vi "Main.vi"() -> ()   [LabVIEW 2020]
doc: "This Continuous Measurement sample project is based on the Queued Message Handler template.\n\nThe Event Handling Loop generates messages based on user interface actions.\n\nThe Message Handling Loop processes messages generated by the Event Handling Loop, or by other messages. There are also Acquisition and Logging message handling loop subVIs, and a chart updating loop."
uses:
  Settings/Settings.ctl
  Acquisition/Hardware Configuration.ctl
  Logging/Logging Configuration.ctl
  controls/UI Data.ctl
  controls/UI State.ctl
  support/Message Queue/Enqueue Message (Single).vi
  <vilib>/Utility/error.llb/Error Cluster From Error Code.vi
  <vilib>/ErrorRing/Error Ring.xnode
  Acquisition/Acquisition.lvlib
  Logging/Logging.lvlib
  Settings/Settings.lvlib
  support/User Event - Stop/User Event - Stop.lvlib
  support/Message Queue/Message Queue.lvlib
  2840X Software Library/Copy of BK PRECISION 2840 Folder/Copy of BK PRECISION 2840.lvlib
  Settings/Settings Dialog.vi
panel:
  in  "Stat In":T1
  out "Tab Ref":refnum<vi>
  out "Trigger Ref":refnum<vi>
  out "COMP Ref":refnum<vi>
  in  "Disconnect":bool
  in  "Connect":bool=TRUE
  out "BIN NO. Ref":refnum<vi>
  out "BIN No.State":bool
  out "BIN State Value":i32
  out "Tolerance New Val":dbl
  out "% Tolerance Ref":refnum<vi>
  out "Nom New Val":dbl
  out "Nominal REF":refnum<vi>
  out "BIN Event Ref":refnum<vi>
  out "Stat Ref":refnum<vi>
  out "Meas Ctl":refnum<vi>
  in  "Meas Tab":enum32{"Measure"}(tab)
  in  "Manual Range":u16(ring)=4 items=["20 m ", "200 m", "2", "20", "200", "2 K", "20 K", "100 K", "1 M", "10 M", "100 M"]
  in  "Auto Range":bool=TRUE
  in  "Function":i32(ring) items=["Resistance", "Resistance and Temperature", "Temperature", "LPR", "LPRT"]
  in  "Aperture":i32(ring)=2 items=["FAST", "MED", "SLOW1", "SLOW2"]
  in  "Average Readings":i32=1 min=1 max=255 step=10
  in  "Trigger Source":u16(ring) items=["Internal", "Manual", "External", "Software (Bus)"]
  in  "Auto Delay":bool=TRUE
  in  "Manual Trigger Delay":dbl=5.0 min=0.0 max=9.999 step=1.0
  in  "Trigger 2":bool
  out "Res":dbl format="%#_6p"
  out "Temp":dbl
  out "Function":string
  out "Meas Color Box":u32(colorbox)=11347 caption="Color Box"
  in  "Tab Control":enum32{"Statistics", "BIN", "Comparator"}(tab)
  out "In Samlpe Count":i32 format="%.0p"
  out "Sample Count":i32 format="%.0p"
  out "MAX":dbl format="%#_6p"
  out "MAX Index":i32 format="%.0p"
  out "MIN":dbl format="%#_6p"
  out "MIN Index":i32 format="%.0p"
  out "HIGH":i32 format="%.0p"
  out "IN":i32 format="%.0p"
  out "LOW":i32 format="%.0p"
  out "MEAS Error":i32 format="%.0p"
  out "Deviation":dbl format="%#_6p"
  out "Variance":dbl format="%#_6p"
  out "Cp":dbl format="%#_6p"
  out "Cpk":i32 format="%.0p"
  in  "Trigger":bool
  in  "Trigger Count":i32=1 min=1 max=250
  in  "Statistics Clear":bool
  in  "Deviation":dbl caption="% Deviation" min=0.0 max=99.999 step=1.0 format="%#_6p"
  in  "Nominal":dbl min=0.0 max=2200000.0 step=1000.0 format="%#_6p"
  in  "State":bool
  in  "Statistics Mode":u16(ring) items=["Percent Error", "Absolute"]
  out "Mean":dbl format="%#_6p"
  out "Stat Color Box":u32(colorbox)=3684408 caption="Color Box"
  in  "BIN State":bool caption="State"
  in  "Beeper Mode":u16(ring) items=["Off", "Beep when Pass", "Beep when Failed"]
  in  "BIN Mode":u16(ring) items=["Tolerance", "Absolute"]
  in  "% Tolerance":T2={"BIN 1"=1.0, "BIN 2"=1.0, "BIN 3"=1.0, "BIN 4"=1.0, "BIN 5"=1.0, "BIN 6"=1.0, "BIN 7"=1.0, "BIN 8"=1.0, "BIN 9"=1.0, "BIN 10"=1.0} {"BIN 10" min=1.0 step=100.0 format="%#_6p"; "BIN 9" min=1.0 step=100.0 format="%#_6p"; "BIN 8" min=1.0 step=100.0 format="%#_6p"; "BIN 7" min=1.0 step=100.0 format="%#_6p"; "BIN 6" min=1.0 step=100.0 format="%#_6p"; "BIN 5" min=1.0 step=100.0 format="%#_6p"; "BIN 4" min=1.0 step=100.0 format="%#_6p"; "BIN 3" min=1.0 step=100.0 format="%#_6p"; "BIN 2" min=1.0 step=100.0 format="%#_6p"; "BIN 1" min=1.0 step=100.0 format="%#_6p"}
  in  "Nominal":T2 {"BIN 10" step=100.0 format="%#_6p"; "BIN 9" step=100.0 format="%#_6p"; "BIN 8" step=100.0 format="%#_6p"; "BIN 7" step=100.0 format="%#_6p"; "BIN 6" step=100.0 format="%#_6p"; "BIN 5" step=100.0 format="%#_6p"; "BIN 4" step=100.0 format="%#_6p"; "BIN 3" step=100.0 format="%#_6p"; "BIN 2" step=100.0 format="%#_6p"; "BIN 1" step=100.0 format="%#_6p"}
  in  "BIN No.":T3
  out "BIN Display":T3
  in  "Comparator Lower":dbl caption="% Tolerance" min=0.0 max=2200000.0 step=1000.0 format="%#_6p"
  in  "Comparator Upper":dbl caption="Nominal" min=0.0 max=2200000.0 step=1000.0 format="%#_6p"
  in  "Comparator Clear":bool
  in  "Comparator Mode":u16(ring) items=["Percent Error", "Absolute"]
  in  "Comparator Beeper":u16(ring) items=["OFF", "NG", "GD"]
  in  "COMP State":bool caption="State"
  out "Comp":string
  out "HI :":i32
  out "LO :":i32
  out "IN :":i32
  out "TOT :":i32
  out "Color Box 3":u32(colorbox)=3684408 caption="Color Box"
  out "Model":string
  out "SN":string
  out "FW Ver.":string
  in  "Settings":bool
  in  "Start":bool
  in  "Stop":bool
  out "Status":string
  in  "Exit":bool
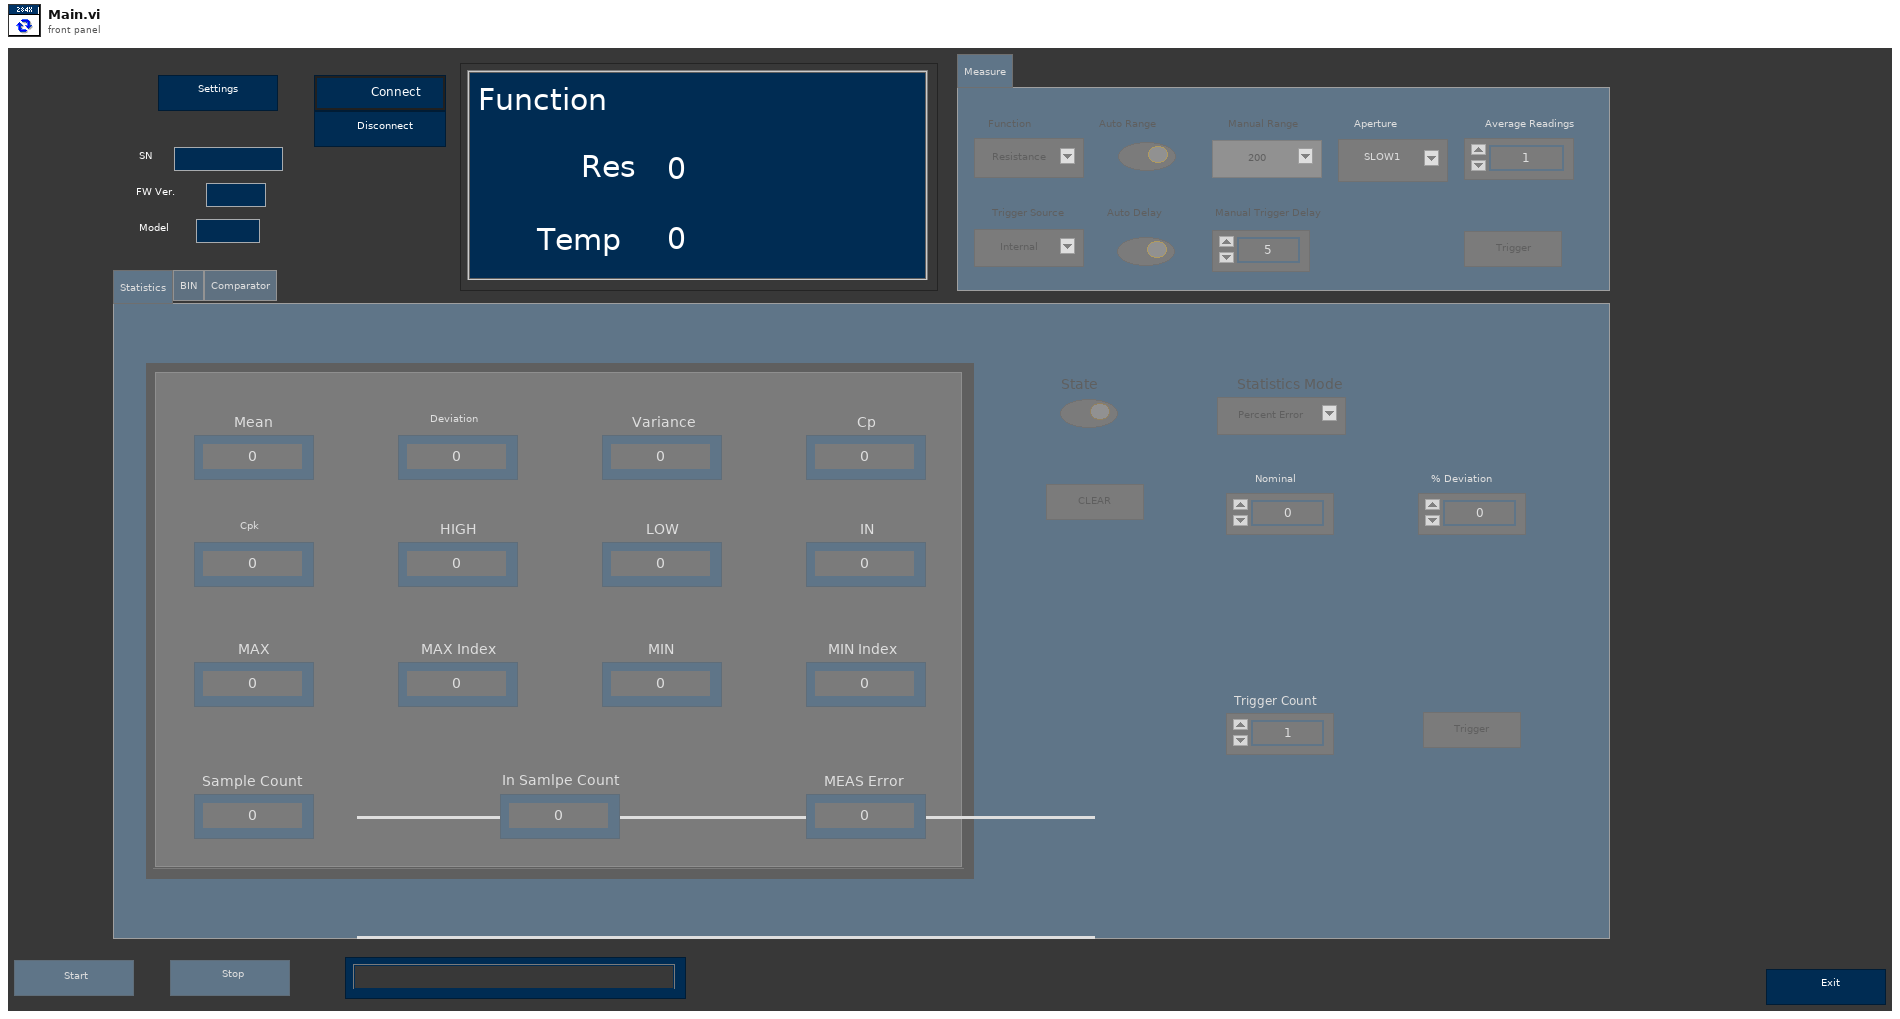
[diagram p1: front panel]
types:
  T1 = cluster{"Sample Count":i32, "IN Sample Count":i32, "Mean":dbl, "MAX":dbl, "MAX Index":i32, "MIN":dbl, "MIN Index":i32, "HIGH":i32, "IN":i32, "LOW":i32, "MEAS Error":i32, "Deviation":dbl, "Variance":dbl, "Cp":dbl, "CpK":i32}
  T2 = cluster{"BIN 1":dbl, "BIN 2":dbl, "BIN 3":dbl, "BIN 4":dbl, "BIN 5":dbl, "BIN 6":dbl, "BIN 7":dbl, "BIN 8":dbl, "BIN 9":dbl, "BIN 10":dbl}
  T3 = cluster{"BIN 1":bool, "BIN 2":bool, "BIN 3":bool, "BIN 4":bool, "BIN 5":bool, "BIN 6":bool, "BIN 7":bool, "BIN 8":bool, "BIN 9":bool, "BIN 10":bool}
  T4 = cluster{"Resistance":dbl, "Temp":dbl, "Function":string}
  T5 = cluster{"Result":string, "Total":i32, " IN":i32, "High":i32, "Low":i32}
  T6 = typedef "UI State.ctl" = enum16{"Idle", "Acquiring and Logging", "Waiting for Exit", "Waiting for Exit (Acq Stopped)", "Waiting for Exit (Log Stopped)", "Waiting for Stop", "Waiting for Stop (Acq Stopped)", "Waiting for Stop (Log Stopped)"}
  T7 = typedef "UI Data.ctl" = cluster{"Start Ref":refnum<vi>, "Stop Ref":refnum<vi>, "Settings Ref":refnum<vi>, "Exit Ref":refnum<vi>, "Status Ref":refnum<vi>, "Meas Trig":refnum<vi>, "Stat Trig":refnum<vi>, "COMP Trig":refnum<vi>, "COMP Mode":refnum<vi>, "COMP Beeper":refnum<vi>, "COMP  Tol":refnum<vi>, "COMP  Nom":refnum<vi>}
  T8 = typedef "Settings.lvlib/Settings.ctl" = cluster{"Hardware Configuration":T9, "Logging Configuration":T10}
  T9 = typedef "Acquisition.lvlib/Hardware Configuration.ctl" = cluster{"Inst.":refnum<visa-resource-name>, "Serial Configuration":cluster{"Baud Rate":u32, "Parity":u16, "Data Bits":u16, "Stop Bits":u16, "Flow Control":u16}, "Reset":bool, "Trigger Count":i32, "BIN State":bool, "COMP State":bool, "Trigger Source":u16, "Stat State ":bool}
  T10 = typedef "Logging.lvlib/Logging Configuration.ctl" = cluster{"*IDN?":string, "File Path":path, "File Path Ref":refnum<file>}
  T11 = typedef "Message Queue.lvlib/All Message Queues.ctl" = cluster{"UI":refnum<queue>, "Acquisition":refnum<queue>, "Logging":refnum<queue>}
  T12 = enum8{"Enabled", "Disabled", "Disabled and Grayed Out"}
  T13 = cluster{"Baud Rate":u32, "Parity":u16, "Data Bits":u16, "Stop Bits":u16, "Flow Control":u16}
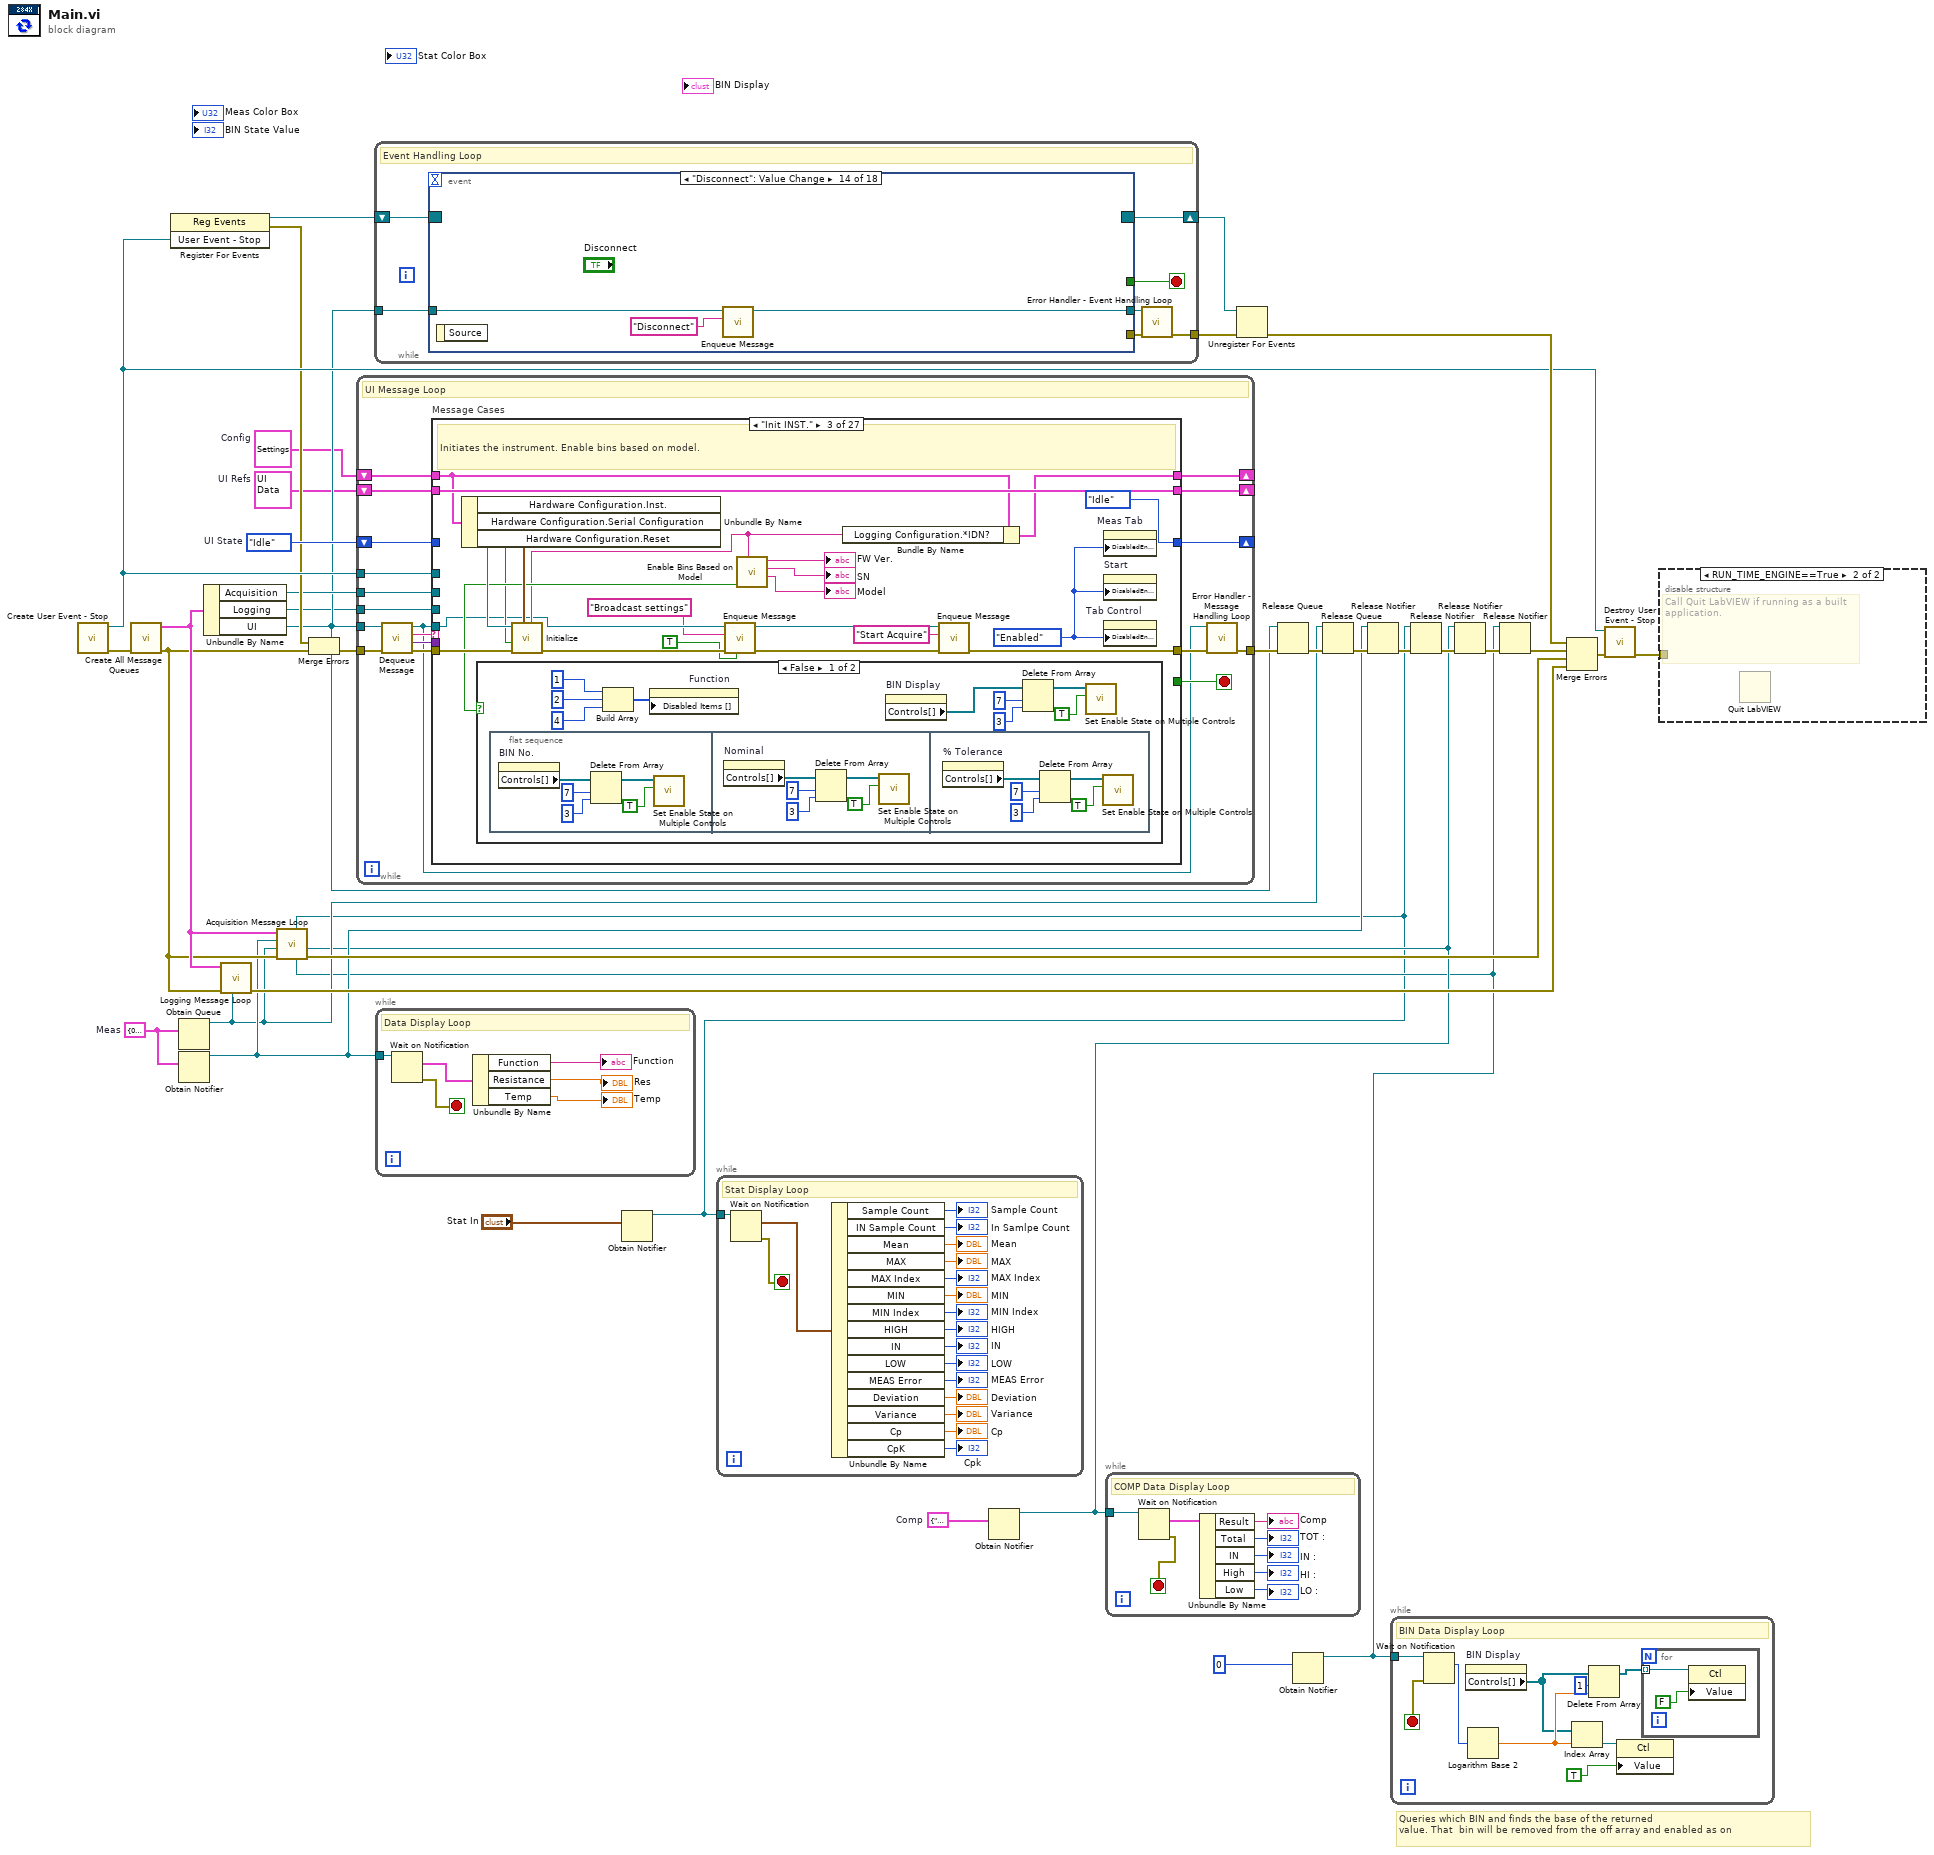
[diagram p0: block diagram]
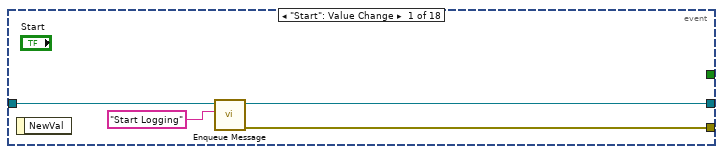
[diagram p3: hidden frame]
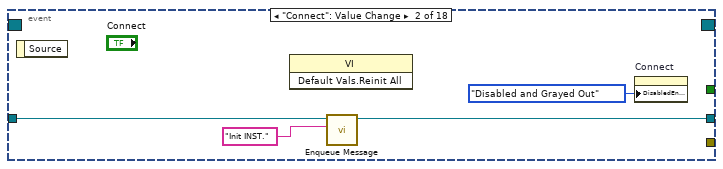
[diagram p4: hidden frame]
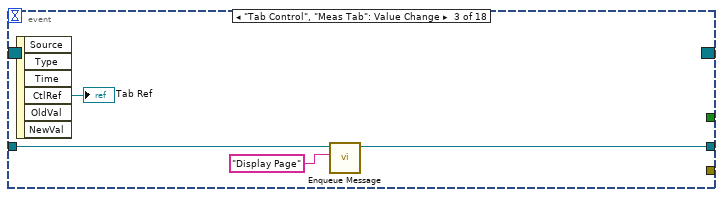
[diagram p5: hidden frame]
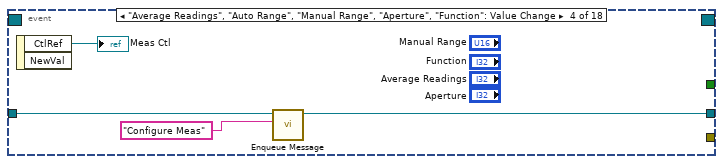
[diagram p6: hidden frame]
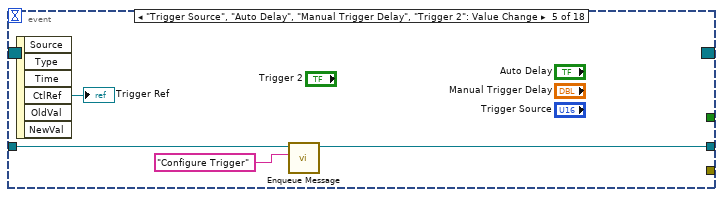
[diagram p7: hidden frame]
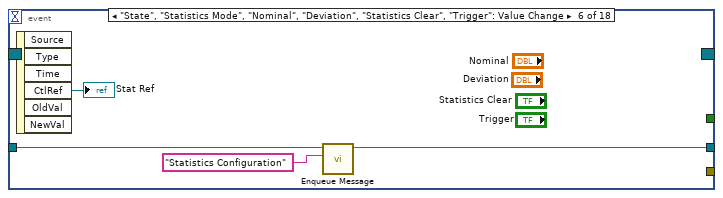
[diagram p8: hidden frame]
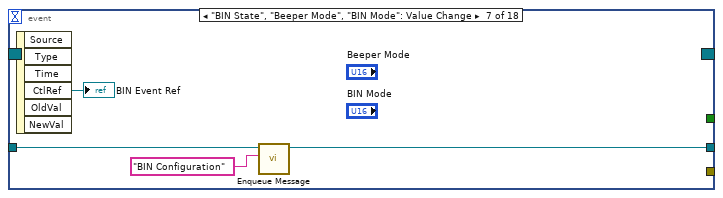
[diagram p9: hidden frame]
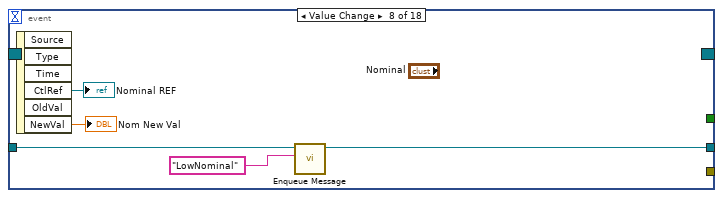
[diagram p10: hidden frame]
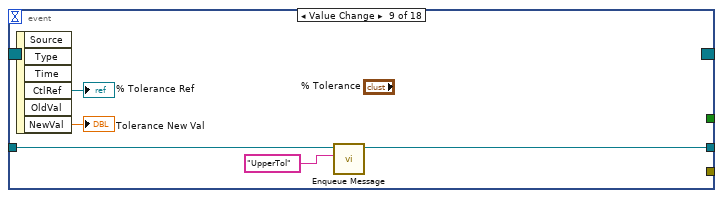
[diagram p11: hidden frame]
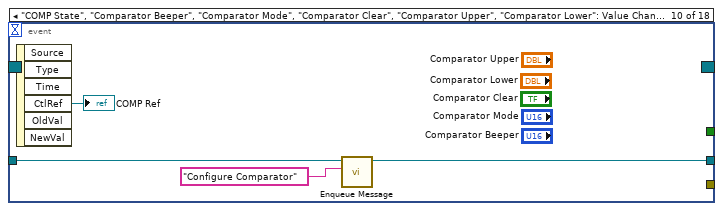
[diagram p12: hidden frame]
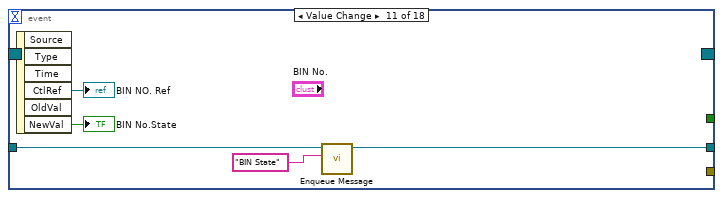
[diagram p13: hidden frame]
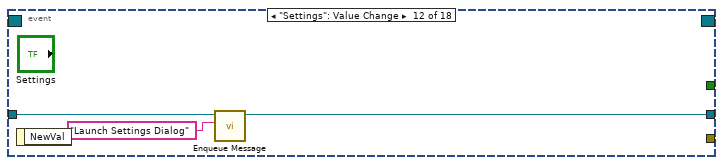
[diagram p14: hidden frame]
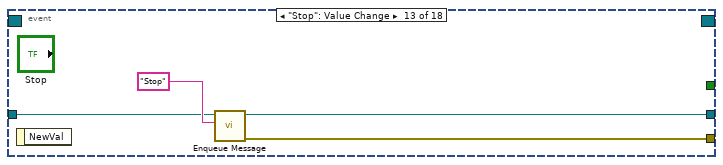
[diagram p15: hidden frame]
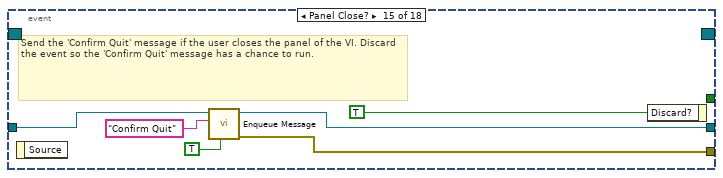
[diagram p16: hidden frame]
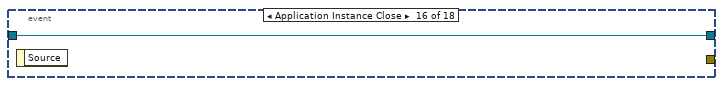
[diagram p17: hidden frame]
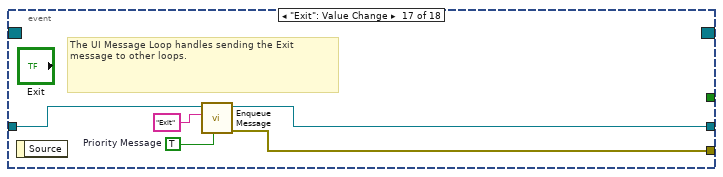
[diagram p18: hidden frame]
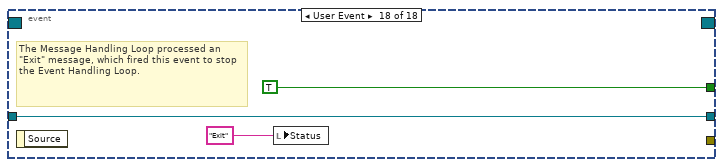
[diagram p19: hidden frame]
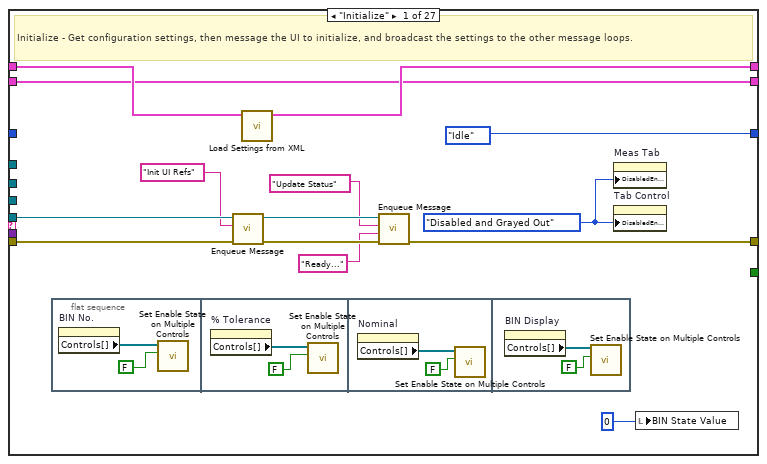
[diagram p20: hidden frame]
diagram:
  w1 = T4 {"Resistance"=0.0, "Temp"=0.0, "Function"=""}  # Meas
  w10 = T5 {"Result"="", "Total"=0, " IN"=0, "High"=0, "Low"=0}  # Comp
  w27 = UI_State."Idle"  # UI State
  w15 = T7 {"Start Ref"=refnum, "Stop Ref"=refnum, "Settings Ref"=refnum, "Exit Ref"=refnum, "Status Ref"=refnum, "Meas Trig"=refnum, "Stat Trig"=refnum, "COMP Trig"=refnum, "COMP Mode"=refnum, "COMP Beeper"=refnum, "COMP  Tol"=refnum, "COMP  Nom"=refnum}  # UI Refs
  w14 = T8 {"Hardware Configuration"={"Inst."="", "Serial Configuration"={"Baud Rate"=0, "Parity"=0, "Data Bits"=8, "Stop Bits"=10, "Flow Control"=0}, "Reset"=FALSE, "Trigger Count"=1, "BIN State"=FALSE, "COMP State"=FALSE, "Trigger Source"=0, "Stat State "=FALSE}, "Logging Configuration"={"*IDN?"="", "File Path"=path "", "File Path Ref"=refnum}}  # Config
  # "Queries which BIN and finds the base of the returned\nvalue. That  bin will be removed from the off array and enabled as on"
  n1 = call "Create User Event - Stop.vi"() -> ("error out"=w33:errorcluster, "User Event - Stop"=w21:refnum<user-event>)  [unwired: 10 in]
  n2 = call "Create All Message Queues.vi"("error in (no error)"=w33) -> ("error out"=w30:errorcluster, "Message Queues out"=w32:T11)  [unwired: 9 in]
  n3 = register-events(w21) -> (reference out=w22:refnum<event-registration>, error out=w19:errorcluster)  [unwired: 2 in]
  n4 = Obtain Queue(element data type=w1) -> (queue out=w12:refnum<queue>)  [unwired: 4 in, 2 out]
  n5 = Obtain Notifier(notification data type=w1) -> (notifier out=w13:refnum<notifier>)  [unwired: 3 in, 2 out]
  n6 = Unbundle By Name(w32) -> ("Acquisition"=w18:refnum<queue>, "Logging"=w16:refnum<queue>, "UI"=w17:refnum<queue>)
  n7 = call "Logging Message Loop.vi"("Meas Queue"=w12, "error in (no error)"=w30, "Message Queues"=w32) -> ("error out"=w31:errorcluster)  [unwired: 8 in]
  n8 = Merge Errors(w19, w30) -> (w20:errorcluster)
  n9 = while {
    tunnel: w17 -> [w48]
    tunnel: w21 -> [w53]
    shift-right: [w47] -> _
    shift-left: w14 -> [w46]
    shift-right: [w44] -> _
    shift-left: w15 -> [w45]
    tunnel: w18 -> [w43]
    tunnel: w16 -> [w42]
    shift-right: [w37] -> _
    shift-left: w27 -> [w38]
    tunnel: w20 -> [w52]
    tunnel: [w41] -> w36
    stop <- w54 stop-if-true
    # "UI Message Loop"
    n10 = call "Dequeue Message.vi"("error in (no error)"=w52, "Message Queue"=w48) -> ("error out"=w51:errorcluster, "Message Data"=w49:variant, "Message"=w50:string, "dup Message Queue"=w39:refnum<queue>)  [unwired: 6 in]
    n11 = case "Message Cases" shown="\"Init INST.\"" w50 {
      selector: w50 -> [_ _ _ _ _ _ _ _ _ _ _ _ _ _ _ _ _ _ _ _ _ _ _ _ _ _ w1131]
      tunnel: w39 -> [w60 _ w102 _ _ w254 w309 _ w415 _ _ _ w810 _ w926 w937 _ w958 w992 w1014 w1040 _ _ w1084 _ _ _]
      tunnel: w51 -> [w59 w83 w114 w159 w198 w260 w316 w411 w425 w475 w619 w761 w817 w907 w925 w936 w953 w959 w993 _ w1042 w1049 w1066 w1083 w1113 w1129 _]
      tunnel: [w64 w83 w105 w158 w199 w259 w315 w410 w424 w474 w618 w765 w816 w900 w909 w929 w940 w956 w990 w1015 w1035 w1053 w1063 w1082 w1123 w1129 w1130] -> w40
      tunnel: [_ _ _ _ _ _ _ _ _ _ _ _ _ _ _ _ _ _ _ _ _ _ _ _ TRUE _ _] -> w54
      tunnel: w49 -> [_ _ _ _ _ _ _ _ _ _ _ _ _ w906 _ _ _ _ _ _ _ w1052 _ _ w1111 _ _]
      tunnel: w53 -> [_ _ _ _ _ _ _ _ _ _ _ _ _ _ _ _ _ _ _ _ _ _ _ _ w1124 _ _]
      tunnel: [w67 w97 w112 w155 w203 w255 w310 w414 w416 w472 w616 w757 w811 w903 w924 w935 w952 w962 w995 w1025 w1039 w1056 w1072 w1087 w1122 w1128 w1134] -> w47
      tunnel: w46 -> [w68 w97 w113 w155 w203 w256 w311 w414 w417 w472 w616 w757 w812 w903 w924 w935 w952 w962 w995 w1025 w1043 w1056 w1072 w1087 w1122 w1128 w1134]
      tunnel: w45 -> [w61 w96 w119 w160 w204 w263 w317 w413 w426 w477 w620 w767 w809 w902 w921 w932 w951 w961 w981 w1023 w1037 w1055 w1071 w1086 w1121 w1127 w1133]
      tunnel: [w61 w94 w119 w160 w204 w263 w317 w413 w426 w477 w620 w767 w809 w902 w921 w932 w951 w961 w981 w1023 w1037 w1055 w1071 w1086 w1121 w1127 w1133] -> w44
      tunnel: w43 -> [_ _ _ w152 _ w253 _ w409 _ _ _ _ _ _ _ w928 _ _ _ w1021 _ _ w1064 _ w1120 _ _]
      tunnel: w42 -> [_ _ _ _ _ _ _ _ _ _ _ _ _ _ w910 _ w941 _ _ w1020 _ _ w1065 _ w1119 _ _]
      tunnel: w38 -> [_ _ _ w157 w195 w257 _ w408 w420 w470 w613 w759 w813 w901 _ w927 w938 w960 w994 w1022 w1036 w1051 w1059 w1085 _ w1126 w1132]
      tunnel: [UI_State."Idle" ("UI State") UI_State."Idle" ("UI State") UI_State."Idle" ("UI State") w157 w195 w257 w312 w408 w420 w470 w613 w759 w813 w901 UI_State."Acquiring and Logging" ("UI State") w927 w939 w957 w991 w1022 w1036 w1051 w1059 w1081 UI_State."Idle" ("UI State") w1126 w1132] -> w37
      frame "Initialize" {
        w55 = T12."Disabled and Grayed Out" ("Disabled")
        # "Initialize - Get configuration settings, then message the UI to initialize, and broadcast the settings to the other message loops."
        n12 = flat-sequence {
          frame #0 {
            n13 = property on="BIN No." class="Clust (strict)"() -> ("Controls[]"=w69:refnum<vi>[])  [unwired: 2 in, 2 out]
            n14 = call "Set Enable State on Multiple Controls.vi"("Enable?"=FALSE, "Controls"=w69) -> ()  [unwired: 10 in]
          }
          frame #1 {
            n15 = property on="% Tolerance" class="Clust (strict)"() -> ("Controls[]"=w72:refnum<vi>[])  [unwired: 2 in, 2 out]
            n16 = call "Set Enable State on Multiple Controls.vi"("Enable?"=FALSE, "Controls"=w72) -> ()  [unwired: 10 in]
          }
          frame #2 {
            n17 = property on="Nominal" class="Clust (strict)"() -> ("Controls[]"=w74:refnum<vi>[])  [unwired: 2 in, 2 out]
            n18 = call "Set Enable State on Multiple Controls.vi"("Enable?"=FALSE, "Controls"=w74) -> ()  [unwired: 10 in]
          }
          frame #3 {
            n19 = property on="BIN Display" class="Clust (strict)"() -> ("Controls[]"=w75:refnum<vi>[])  [unwired: 2 in, 2 out]
            n20 = call "Set Enable State on Multiple Controls.vi"("Enable?"=FALSE, "Controls"=w75) -> ()  [unwired: 10 in]
          }
        }
        n21 = call-poly "Enqueue Message.vi"("error in (no error)"=w59, "Message"="Init UI Refs", "Message Queue"=w60) -> ("error out"=w66:errorcluster, "dup Message Queue"=w65:refnum<queue>)  [unwired: 7 in]
        n22 = call "Load Settings from XML.vi"("Settings in"=w68) -> ("Settings out"=w67:T8)  [unwired: 9 in, 1 out]
        n23 = call-poly "Enqueue Message.vi"("error in (no error)"=w66, "Message Data"="Ready..." ("Ready..."), "Message"="Update Status", "Message Queue"=w65) -> ("error out"=w64:errorcluster)  [unwired: 6 in, 1 out]
        n24 = property on="Meas Tab" class="TabCtl (strict)"("DisabledEnum"=w55) -> ()  [unwired: 2 in, 2 out]
        n25 = property on="Tab Control" class="TabCtl (strict)"("DisabledEnum"=w55) -> ()  [unwired: 2 in, 2 out]
        n26 = local write "BIN State Value"(0) -> ()
      }
      frame "Init UI Refs" {
        # "Enable: Start, Exit, Settings\nDisable: Stop"
        # "Init UI Refs - Store control references for UI controls.  Also enable/disable controls appropriately."
        n27 = control-ref of="Comparator Clear"() -> (w82:refnum<vi>)
        n28 = control-ref of="Stat Trig"() -> (w84:refnum<vi>)
        n29 = control-ref of="Meas Trig"() -> (w85:refnum<vi>)
        n30 = control-ref of="Stop"() -> (w86:refnum<vi>)
        n31 = control-ref of="Start"() -> (w77:refnum<vi>)
        n32 = control-ref of="Settings"() -> (w89:refnum<vi>)
        n33 = control-ref of="Exit"() -> (w88:refnum<vi>)
        n34 = control-ref of="Comparator Lower"() -> (w79:refnum<vi>)
        n35 = control-ref of="Comparator Upper"() -> (w78:refnum<vi>)
        n36 = control-ref of="Status"() -> (w95:refnum<vi>)
        n37 = control-ref of="Comparator Mode"() -> (w81:refnum<vi>)
        n38 = control-ref of="Comparator Beeper"() -> (w80:refnum<vi>)
        n39 = Bundle By Name(cluster=w96, "COMP Trig"=w82, "Stat Trig"=w84, "Meas Trig"=w85, "Stop Ref"=w86, "Start Ref"=w77, "Settings Ref"=w89, "Exit Ref"=w88, "Status Ref"=w95, "COMP Mode"=w81, "COMP Beeper"=w80, "COMP  Tol"=w79, "COMP  Nom"=w78) -> (w94:T7)
        n40 = Build Array(w89, w88) -> (w92:refnum<vi>[])
        n41 = Build Array(w84, w85, w86, w77) -> (w91:refnum<vi>[])
        n42 = call "Set Enable State on Multiple Controls.vi"("Enable?"=TRUE, "Controls"=w92) -> ()  [unwired: 10 in]
        n43 = call "Set Enable State on Multiple Controls.vi"("Enable?"=FALSE, "Controls"=w91) -> ()  [unwired: 10 in]
      }
      frame "Init INST." {
        w98 = T12."Enabled" ("Disabled")
        # "Initiates the instrument. Enable bins based on model."
        n44 = Unbundle By Name(w113) -> ("Hardware Configuration.Inst."=w115:refnum<visa-resource-name>, "Hardware Configuration.Serial Configuration"=w116:T13, "Hardware Configuration.Reset"=w108:bool)
        n45 = call "Initialize.vi"("Serial Configuration"=w116, "error in (no error)"=w114, "Reset (True)"=w108, "VISA resource name"=w115) -> ("error out"=w104:errorcluster, "*IDN?"=w107:string)  [unwired: 5 in, 1 out]
        n46 = call-poly "Enqueue Message.vi"("Priority Message? (F)"=TRUE, "error in (no error)"=w104, "Message"="Broadcast settings", "Message Queue"=w102) -> ("error out"=w103:errorcluster, "dup Message Queue"=w99:refnum<queue>)  [unwired: 6 in]
        n47 = call "Enable Bins Based on Model.vi"("*IDN"=w107) -> ("model 2841?"=w110:bool, "Model"=→"Model":string, "SN"=→"SN":string, "FW Ver."=→"FW Ver.":string)  [unwired: 7 in]
        n48 = case shown="False" w110 {
          frame False {
            n49 = flat-sequence {
              frame #0 {
                n50 = property on="BIN No." class="Clust (strict)"() -> ("Controls[]"=w133:refnum<vi>[])  [unwired: 2 in, 2 out]
                n51 = Delete From Array(array=w133, length=7, index=3) -> (array with subset deleted=w130:refnum<vi>[])  [unwired: 1 out]
                n52 = call "Set Enable State on Multiple Controls.vi"("Enable?"=TRUE, "Controls"=w130) -> ()  [unwired: 10 in]
              }
              frame #1 {
                n53 = property on="Nominal" class="Clust (strict)"() -> ("Controls[]"=w138:refnum<vi>[])  [unwired: 2 in, 2 out]
                n54 = Delete From Array(array=w138, length=7, index=3) -> (array with subset deleted=w136:refnum<vi>[])  [unwired: 1 out]
                n55 = call "Set Enable State on Multiple Controls.vi"("Enable?"=TRUE, "Controls"=w136) -> ()  [unwired: 10 in]
              }
              frame #2 {
                n56 = property on="% Tolerance" class="Clust (strict)"() -> ("Controls[]"=w143:refnum<vi>[])  [unwired: 2 in, 2 out]
                n57 = Delete From Array(array=w143, length=7, index=3) -> (array with subset deleted=w141:refnum<vi>[])  [unwired: 1 out]
                n58 = call "Set Enable State on Multiple Controls.vi"("Enable?"=TRUE, "Controls"=w141) -> ()  [unwired: 10 in]
              }
            }
            n59 = Build Array(1, 2, 4) -> (w125:i32[])
            n60 = property on="Function" class="Ring (strict)"("Disabled Items []"=w125) -> ()  [unwired: 2 in, 2 out]
            n61 = property on="BIN Display" class="Clust (strict)"() -> ("Controls[]"=w124:refnum<vi>[])  [unwired: 2 in, 2 out]
            n62 = Delete From Array(array=w124, length=7, index=3) -> (array with subset deleted=w122:refnum<vi>[])  [unwired: 1 out]
            n63 = call "Set Enable State on Multiple Controls.vi"("Enable?"=TRUE, "Controls"=w122) -> ()  [unwired: 10 in]
          }
          frame True {
            n64 = flat-sequence {
              frame #0 {
                n65 = property on="BIN No." class="Clust (strict)"() -> ("Controls[]"=w144:refnum<vi>[])  [unwired: 2 in, 2 out]
                n66 = call "Set Enable State on Multiple Controls.vi"("Enable?"=TRUE, "Controls"=w144) -> ()  [unwired: 10 in]
              }
              frame #1 {
                n67 = property on="Nominal" class="Clust (strict)"() -> ("Controls[]"=w147:refnum<vi>[])  [unwired: 2 in, 2 out]
                n68 = call "Set Enable State on Multiple Controls.vi"("Enable?"=TRUE, "Controls"=w147) -> ()  [unwired: 10 in]
              }
              frame #2 {
                n69 = property on="% Tolerance" class="Clust (strict)"() -> ("Controls[]"=w149:refnum<vi>[])  [unwired: 2 in, 2 out]
                n70 = call "Set Enable State on Multiple Controls.vi"("Enable?"=TRUE, "Controls"=w149) -> ()  [unwired: 10 in]
              }
              frame #3 {
                n71 = property on="BIN Display" class="Clust (strict)"() -> ("Controls[]"=w151:refnum<vi>[])  [unwired: 2 in, 2 out]
                n72 = call "Set Enable State on Multiple Controls.vi"("Enable?"=TRUE, "Controls"=w151) -> ()  [unwired: 10 in]
              }
            }
          }
        }
        n73 = Bundle By Name(cluster=w113, "Logging Configuration.*IDN?"=w107) -> (w112:T8)
        n74 = call-poly "Enqueue Message.vi"("error in (no error)"=w103, "Message"="Start Acquire", "Message Queue"=w99) -> ("error out"=w105:errorcluster)  [unwired: 7 in, 1 out]
        n75 = property on="Meas Tab" class="TabCtl (strict)"("DisabledEnum"=w98) -> ()  [unwired: 2 in, 2 out]
        n76 = property on="Start" class="Bool"("DisabledEnum"=w98) -> ()  [unwired: 2 in, 2 out]
        n77 = property on="Tab Control" class="TabCtl (strict)"("DisabledEnum"=w98) -> ()  [unwired: 2 in, 2 out]
      }
      frame "Display Page" {
        # "Sets the display page on the instrument based on the selected tab."
        n78 = Unbundle By Name(w155) -> ("Hardware Configuration.Inst."=w156:refnum<visa-resource-name>)
        n79 = local read "Tab Ref"() -> (w154:refnum<vi>)
        n80 = property class="TabCtl"(reference=w154) -> ("Label.Text"=w153:string)  [unwired: 1 in, 2 out]
        n81 = case shown="\"Tab Control\"" w153 {
          tunnel: w159 -> [w161 w167 w194]
          tunnel: [w161 w166 w194] -> w158
          tunnel: w156 -> [_ w165 _]
          tunnel: w152 -> [_ w163 _]
          frame "False", Default {
          }
          frame "Tab Control" {
            n82 = case shown="\"BIN\"" "Tab Control" {
              tunnel: w167 -> [w172 w184 w188]
              tunnel: [w176 w183 w193] -> w166
              tunnel: w165 -> [w174 w181 w191]
              tunnel: w163 -> [w173 w180 w186]
              tunnel: TRUE -> [w168 w177 w185]
              frame "Statistics", Default {
                n83 = call-poly "Enqueue Message.vi"("Priority Message? (F)"=w168, "error in (no error)"=w172, "Message Data"="Stat" ("Message"), "Message"="Display Page Change", "Message Queue"=w173) -> ("error out"=w171:errorcluster)  [unwired: 5 in, 1 out]
                n84 = call "Write.vi"("Input String"=":DISP:PAGE STAT;", "error in (no error)"=w171, "VISA resource name"=w174) -> ("error out"=w176:errorcluster)  [unwired: 7 in, 1 out]
              }
              frame "BIN" {
                n85 = call-poly "Enqueue Message.vi"("Priority Message? (F)"=w177, "Message Data"="BIN" ("Message"), "Message"="Display Page Change", "Message Queue"=w180) -> ()  [unwired: 6 in, 2 out]
                n86 = call "Write.vi"("Input String"=":DISP:PAGE BIN;", "error in (no error)"=w184, "VISA resource name"=w181) -> ("error out"=w183:errorcluster)  [unwired: 7 in, 1 out]
              }
              frame "Comparator" {
                n87 = call-poly "Enqueue Message.vi"("Priority Message? (F)"=w185, "error in (no error)"=w188, "Message Data"="COMP" ("Message"), "Message"="Display Page Change", "Message Queue"=w186) -> ("error out"=w187:errorcluster)  [unwired: 5 in, 1 out]
                n88 = call "Write.vi"("Input String"=":DISP:PAGE COMP;", "error in (no error)"=w187, "VISA resource name"=w191) -> ("error out"=w193:errorcluster)  [unwired: 7 in, 1 out]
              }
            }
          }
          frame "Meas Tab" {
          }
        }
      }
      frame "Configure Meas" {
        # "Configure the function, Auto Range state, or the Manual Range."
        n89 = local read "Meas Ctl"() -> (w202:refnum<vi>)
        n90 = Unbundle By Name(w203) -> ("Hardware Configuration.Inst."=w197:refnum<visa-resource-name>)
        n91 = local read "Function"() -> (w200:i32)
        n92 = property class="Ctl"(reference=w202) -> ("Label.Text"=w201:string)  [unwired: 1 in, 2 out]
        n93 = case shown="\"Function\"" w201 {
          tunnel: w200 -> [_ w210 w225 w237 _ _]
          tunnel: [w205 w208 w222 w232 w243 w248] -> w199
          tunnel: w198 -> [w205 w207 w215 w231 w242 w249]
          tunnel: w197 -> [_ w206 w221 w230 w241 w247]
          tunnel: "Auto Range" -> [_ _ w214 _ _ _]
          frame "False", Default {
          }
          frame "Function" {
            w213 = ":FUNC:IMP %s;"  # Select Function
            n94 = Pick Line(multi-line string=" R\nRT\nT\nLPR\nLPRT", line index=w210) -> (output string=w211:string)  [unwired: 1 in]
            n95 = Format Into String(format string=w213, w211) -> (resulting string=w209:string)  [unwired: 2 in, 1 out]
            n96 = call "Write.vi"("Input String"=w209, "error in (no error)"=w207, "VISA resource name"=w206) -> ("error out"=w208:errorcluster)  [unwired: 7 in, 1 out]
          }
          frame "Auto Range" {
            w218 = "%;:FUNC:IMP:%s:RANG:AUTO 1;"  # Auto Range
            w223 = "%;:FUNC:IMP:%s:RANG:AUTO 0;"  # Manual Range
            n97 = Pick Line(multi-line string="RES\nRES\nRES\nLPR\nLPR", line index=w225) -> (output string=w217:string)  [unwired: 1 in]
            n98 = Format Into String(format string=w218, w217) -> (resulting string=w216:string)  [unwired: 2 in, 1 out]
            n99 = Format Into String(format string=w223, w217) -> (resulting string=w219:string)  [unwired: 2 in, 1 out]
            n100 = case shown="False" w214 {
              frame False {
                n101 = property on="Manual Range" class="Ring (strict)"("DisabledEnum"=T12."Enabled" ("Disabled")) -> ()  [unwired: 2 in, 2 out]
              }
              frame True {
                n102 = property on="Manual Range" class="Ring (strict)"("DisabledEnum"=T12."Disabled and Grayed Out" ("Disabled")) -> ()  [unwired: 2 in, 2 out]
              }
            }
            n103 = Select(t=w216, s=w214, f=w219) -> (s? t:f=w220:string)
            n104 = call "Write.vi"("Input String"=w220, "error in (no error)"=w215, "VISA resource name"=w221) -> ("error out"=w222:errorcluster)  [unwired: 7 in, 1 out]
          }
          frame "Manual Range" {
            w236 = "%.;:FUNC:IMP:%s:RANG %s;"  # Manual Range
            n105 = local read "Manual Range"() -> (w228:u16)
            n106 = Pick Line(multi-line string="RES\nRES\nRES\nLPR\nLPR", line index=w237) -> (output string=w234:string)  [unwired: 1 in]
            n107 = Pick Line(multi-line string=".02 \n .2\n2\n20\n200\n2000\n20000\n100000\n1000000\n10000000\n100000000", line index=w228) -> (output string=w233:string)  [unwired: 1 in]
            n108 = Format Into String(format string=w236, w234, w233) -> (resulting string=w229:string)  [unwired: 2 in, 1 out]
            n109 = call "Write.vi"("Input String"=w229, "error in (no error)"=w231, "VISA resource name"=w230) -> ("error out"=w232:errorcluster)  [unwired: 7 in, 1 out]
          }
          frame "Average Readings" {
            w244 = ":APER:AVER %d;"  # Select Aperture
            n110 = local read "Average Readings"() -> (w239:i32)
            n111 = Format Into String(format string=w244, w239) -> (resulting string=w240:string)  [unwired: 2 in, 1 out]
            n112 = call "Write.vi"("Input String"=w240, "error in (no error)"=w242, "VISA resource name"=w241) -> ("error out"=w243:errorcluster)  [unwired: 7 in, 1 out]
          }
          frame "Aperture" {
            w251 = ":APER %s;"  # Select Aperture
            n113 = local read "Aperture"() -> (w245:i32)
            n114 = Pick Line(multi-line string="FAST\nMED\nSLOW1\nSLOW2", line index=w245) -> (output string=w252:string)  [unwired: 1 in]
            n115 = Format Into String(format string=w251, w252) -> (resulting string=w246:string)  [unwired: 2 in, 1 out]
            n116 = call "Write.vi"("Input String"=w246, "error in (no error)"=w249, "VISA resource name"=w247) -> ("error out"=w248:errorcluster)  [unwired: 7 in, 1 out]
          }
        }
      }
      frame "Configure Trigger" {
        # "Configure the triggers settings (Source, Auto Delay, Manual Delay.)"
        n117 = Unbundle By Name(w256) -> ("Hardware Configuration.Inst."=w258:refnum<visa-resource-name>)
        n118 = local read "Trigger Ref"() -> (w262:refnum<vi>)
        n119 = property class="Ctl"(reference=w262) -> ("Label.Text"=w261:string)  [unwired: 1 in, 2 out]
        n120 = case shown="\"Trigger Source\"" w261 {
          tunnel: w260 -> [w265 w275 w294 w301 w306]
          tunnel: [w265 w283 w293 w300 w305] -> w259
          tunnel: w258 -> [_ w278 w292 w299 _]
          tunnel: w256 -> [w264 w277 w284 w295 w303]
          tunnel: [w264 w276 w284 w295 w303] -> w255
          tunnel: w254 -> [_ w273 _ _ _]
          tunnel: w253 -> [_ _ _ _ w302]
          frame "False", Default {
          }
          frame "Trigger Source" {
            w282 = "INT;\nMAN;\nEXT;\nBUS;"  # Trigger Source
            n121 = local read "Trigger Source"() -> (w271:u16)
            n122 = Bundle By Name(cluster=w277, "Hardware Configuration.Trigger Source"=w271) -> (w276:T8)
            n123 = Equal?(x=w271, y=3) -> (x = y?=w269:bool)
            n124 = Select(t=T12."Enabled" ("Disabled"), s=w269, f=T12."Disabled and Grayed Out" ("Disabled")) -> (s? t:f=w266:T12)
            n125 = Pick Line(multi-line string=w282, line index=w271) -> (output string=w280:string)  [unwired: 1 in]
            n126 = call-poly "Enqueue Message.vi"("error in (no error)"=w275, "Message"="Broadcast settings", "Message Queue"=w273) -> ("error out"=w274:errorcluster)  [unwired: 7 in, 1 out]
            n127 = Format Into String(format string=":TRIGger:SOURce %s", w280) -> (resulting string=w279:string)  [unwired: 2 in, 1 out]
            n128 = property on="Trigger 2" class="Bool"("DisabledEnum"=w266) -> ()  [unwired: 2 in, 2 out]
            n129 = property on="Trigger" class="Bool"("DisabledEnum"=w266) -> ()  [unwired: 2 in, 2 out]
            n130 = call "Write.vi"("Input String"=w279, "error in (no error)"=w274, "VISA resource name"=w278) -> ("error out"=w283:errorcluster)  [unwired: 7 in, 1 out]
          }
          frame "Auto Delay" {
            w291 = ":TRIG:DEL:AUTO 0;"  # Disable Auto Delay
            w289 = ":TRIG:DEL:AUTO 1;"  # Enable Auto Delay
            n131 = local read "Auto Delay"() -> (w285:bool)
            n132 = Select(t=T12."Disabled and Grayed Out" ("Disabled"), s=w285, f=T12."Enabled" ("Disabled")) -> (s? t:f=w288:T12)
            n133 = Select(t=w289, s=w285, f=w291) -> (s? t:f=w290:string)
            n134 = call "Write.vi"("Input String"=w290, "error in (no error)"=w294, "VISA resource name"=w292) -> ("error out"=w293:errorcluster)  [unwired: 7 in, 1 out]
            n135 = property on="Manual Trigger Delay" class="DigNum (strict)"("DisabledEnum"=w288) -> ()  [unwired: 2 in, 2 out]
          }
          frame "Manual Trigger Delay" {
            w298 = "%.;:TRIG:DEL %g;"  # Manual Trigger Delay
            n136 = local read "Manual Trigger Delay"() -> (w296:dbl)
            n137 = Format Into String(format string=w298, w296) -> (resulting string=w297:string)  [unwired: 2 in, 1 out]
            n138 = call "Write.vi"("Input String"=w297, "error in (no error)"=w301, "VISA resource name"=w299) -> ("error out"=w300:errorcluster)  [unwired: 7 in, 1 out]
          }
          frame "Trigger 2" {
            n139 = call-poly "Enqueue Message.vi"("error in (no error)"=w306, "Message"="Single Meas", "Message Queue"=w302) -> ("error out"=w305:errorcluster)  [unwired: 7 in, 1 out]
          }
        }
      }
      frame "Statistics Configuration" {
        w312 = UI_State."Idle"  # UI State
        # "Configure or clear the Statistics tab.(State, mode, and limits)"
        n140 = local read "Stat Ref"() -> (w308:refnum<vi>)
        n141 = Unbundle By Name(w311) -> ("Hardware Configuration.Inst."=w314:refnum<visa-resource-name>)
        n142 = property class="Ctl"(reference=w308) -> ("Label.Text"=w307:string)  [unwired: 1 in, 2 out]
        n143 = case shown="\"Trigger\"" w307 {
          tunnel: w316 -> [w319 w323 w352 w361 w379 w402 w407]
          tunnel: [w319 w324 w351 w360 w378 w395 w406] -> w315
          tunnel: w314 -> [_ w336 w349 w359 w377 _ w404]
          tunnel: "Statistics Mode" -> [_ _ w348 w356 w374 _ _]
          tunnel: w311 -> [w318 w327 w347 w358 w376 w401 w403]
          tunnel: [w318 w326 w347 w358 w376 w400 w403] -> w310
          tunnel: w309 -> [_ w320 _ _ _ w398 _]
          frame "False", Default {
          }
          frame "State" {
            n144 = call-poly "Enqueue Message.vi"("error in (no error)"=w323, "Message"="Broadcast settings", "Message Queue"=w320) -> ("error out"=w322:errorcluster)  [unwired: 7 in, 1 out]
            n145 = Select(t=1, s="State", f=0) -> (s? t:f=w334:i32)
            n146 = Bundle By Name(cluster=w327, "Hardware Configuration.Stat State"="State") -> (w326:T8)
            n147 = Format Into String(format string=":STAT %d;", w334) -> (resulting string=w332:string)  [unwired: 2 in, 1 out]
            n148 = call "Write.vi"("Input String"=w332, "error in (no error)"=w322, "VISA resource name"=w336) -> ("error out"=w324:errorcluster)  [unwired: 7 in, 1 out]
            n149 = Select(t=T12."Disabled and Grayed Out" ("Disabled"), s="State", f=T12."Enabled" ("Disabled")) -> (s? t:f=w328:T12)
            n150 = property on="Statistics Clear" class="Bool"("DisabledEnum"=w328) -> ()  [unwired: 2 in, 2 out]
            n151 = property on="Statistics Mode" class="Ring (strict)"("DisabledEnum"=w328) -> ()  [unwired: 2 in, 2 out]
          }
          frame "Statistics Mode" {
            n152 = Pick Line(multi-line string="PTOL\nATOL", line index=w348) -> (output string=w354:string)  [unwired: 1 in]
            n153 = Equal To 0?(x=w348) -> (x = 0?=w339:bool)
            n154 = Format Into String(format string="STAT:MODE %s;" ("true string"), w354) -> (resulting string=w350:string)  [unwired: 2 in, 1 out]
            n155 = call "Write.vi"("Input String"=w350, "error in (no error)"=w352, "VISA resource name"=w349) -> ("error out"=w351:errorcluster)  [unwired: 7 in, 1 out]
            n156 = Select(t="% Deviation", s=w339, f="Lower Limit") -> (s? t:f=w341:string)
            n157 = Select(t="Nominal", s=w339, f="Upper Limit") -> (s? t:f=w343:string)
            n158 = Select(t=99.999, s=w339, f=2200000.0 ("t")) -> (s? t:f=w340:dbl)
            n159 = property on="Deviation" class="DigNum (strict)"("Caption.Text"=w341) -> ()  [unwired: 2 in, 2 out]
            n160 = property on="Nominal" class="DigNum (strict)"("Caption.Text"=w343) -> ()  [unwired: 2 in, 2 out]
            n161 = property on="Deviation" class="DigNum (strict)"("Maximum"=w340) -> ()  [unwired: 2 in, 2 out]
          }
          frame "Nominal" {
            n162 = local read "Nominal"() -> (w357:dbl)
            n163 = case shown="0, Default" w356 {
              tunnel: w361 -> [w367 w370]
              tunnel: [w366 w371] -> w360
              tunnel: w359 -> [w363 w369]
              tunnel: w357 -> [w362 w368]
              frame 0, Default {
                n164 = Format Into String(format string=":STAT:REF %f" ("true string"), w362) -> (resulting string=w364:string)  [unwired: 2 in, 1 out]
                n165 = call "Write.vi"("Input String"=w364, "error in (no error)"=w367, "VISA resource name"=w363) -> ("error out"=w366:errorcluster)  [unwired: 7 in, 1 out]
              }
              frame 1 {
                n166 = Format Into String(format string=":STAT:UPP %f" ("true string"), w368) -> (resulting string=w373:string)  [unwired: 2 in, 1 out]
                n167 = call "Write.vi"("Input String"=w373, "error in (no error)"=w370, "VISA resource name"=w369) -> ("error out"=w371:errorcluster)  [unwired: 7 in, 1 out]
              }
            }
          }
          frame "Deviation" {
            n168 = local read "Deviation"() -> (w375:dbl)
            n169 = case shown="1" w374 {
              tunnel: w379 -> [w385 w389]
              tunnel: [w384 w387] -> w378
              tunnel: w377 -> [w383 w388]
              tunnel: w375 -> [w380 w386]
              frame 0, Default {
                n170 = Format Into String(format string=":STAT:PERC %f;" ("true string"), w380) -> (resulting string=w381:string)  [unwired: 2 in, 1 out]
                n171 = call "Write.vi"("Input String"=w381, "error in (no error)"=w385, "VISA resource name"=w383) -> ("error out"=w384:errorcluster)  [unwired: 7 in, 1 out]
              }
              frame 1 {
                n172 = Format Into String(format string=":STAT:LOW %f" ("true string"), w386) -> (resulting string=w391:string)  [unwired: 2 in, 1 out]
                n173 = call "Write.vi"("Input String"=w391, "error in (no error)"=w389, "VISA resource name"=w388) -> ("error out"=w387:errorcluster)  [unwired: 7 in, 1 out]
              }
            }
          }
          frame "Trigger" {
            n174 = Bundle By Name(cluster=w401, "Hardware Configuration.Trigger Count"="Trigger Count") -> (w400:T8)
            n175 = call-poly "Enqueue Message.vi"("Priority Message? (F)"=TRUE, "error in (no error)"=w402, "Message"="Broadcast settings", "Message Queue"=w398) -> ("error out"=w396:errorcluster, "dup Message Queue"=w392:refnum<queue>)  [unwired: 6 in]
            n176 = call-poly "Enqueue Message.vi"("error in (no error)"=w396, "Message"="Statistic Acquire", "Message Queue"=w392) -> ("error out"=w395:errorcluster)  [unwired: 7 in, 1 out]
          }
          frame "Statistics Clear" {
            n177 = call "Write.vi"("Input String"="STATistics:CLEAr", "error in (no error)"=w407, "VISA resource name"=w404) -> ("error out"=w406:errorcluster)  [unwired: 7 in, 1 out]
          }
        }
      }
      frame "Statistic Acquire" {
        # "Acquire single STAT meas in acquire vi after settings are broadcast."
        n178 = call-poly "Enqueue Message.vi"("error in (no error)"=w411, "Message"="Statistic Acquire", "Message Queue"=w409) -> ("error out"=w410:errorcluster)  [unwired: 7 in, 1 out]
      }
      frame "BIN Configuration" {
        # "Configure the BIN tab.(BIN State,BIN Mode, Beeper Mode)"
        n179 = local read "BIN Event Ref"() -> (w419:refnum<vi>)
        n180 = Unbundle By Name(w417) -> ("Hardware Configuration.Inst."=w423:refnum<visa-resource-name>)
        n181 = local read "Beeper Mode"() -> (w422:u16)
        n182 = local read "BIN Mode"() -> (w421:u16)
        n183 = property class="Ctl"(reference=w419) -> ("Label.Text"=w418:string)  [unwired: 1 in, 2 out]
        n184 = case shown="\"False\", Default" w418 {
          tunnel: w425 -> [w428 w434 w454 w467]
          tunnel: [w428 w440 w453 w466] -> w424
          tunnel: w423 -> [_ w439 w455 w465]
          tunnel: w421 -> [_ _ w451 _]
          tunnel: w422 -> [_ _ _ w460]
          tunnel: w417 -> [w427 w432 w445 w459]
          tunnel: [w427 w430 w445 w459] -> w416
          tunnel: w415 -> [_ w429 _ _]
          frame "False", Default {
          }
          frame "BIN State" {
            n185 = call-poly "Enqueue Message.vi"("error in (no error)"=w434, "Message"="Broadcast settings", "Message Queue"=w429) -> ("error out"=w433:errorcluster)  [unwired: 7 in, 1 out]
            n186 = Bundle By Name(cluster=w432, "Hardware Configuration.BIN State"="BIN State") -> (w430:T8)
            n187 = Select(t=1, s="BIN State", f=0) -> (s? t:f=w441:i32)
            n188 = Format Into String(format string=":BIN %d;", w441) -> (resulting string=w436:string)  [unwired: 2 in, 1 out]
            n189 = call "Write.vi"("Input String"=w436, "error in (no error)"=w433, "VISA resource name"=w439) -> ("error out"=w440:errorcluster)  [unwired: 7 in, 1 out]
          }
          frame "BIN Mode" {
            n190 = Equal To 0?(x=w451) -> (x = 0?=w446:bool)
            n191 = Pick Line(multi-line string="PTOL\nATOL", line index=w451) -> (output string=w456:string)  [unwired: 1 in]
            n192 = Format Into String(format string=":BIN:MODE %s;" ("true string"), w456) -> (resulting string=w452:string)  [unwired: 2 in, 1 out]
            n193 = Select(t="% Tolerance", s=w446, f="Upper Limit") -> (s? t:f=w443:string)
            n194 = Select(t="Nominal", s=w446, f="Lower Limit") -> (s? t:f=w444:string)
            n195 = call "Write.vi"("Input String"=w452, "error in (no error)"=w454, "VISA resource name"=w455) -> ("error out"=w453:errorcluster)  [unwired: 7 in, 1 out]
            n196 = property on="% Tolerance" class="Clust (strict)"("Caption.Text"=w443) -> ()  [unwired: 2 in, 2 out]
            n197 = property on="Nominal" class="Clust (strict)"("Caption.Text"=w444) -> ()  [unwired: 2 in, 2 out]
          }
          frame "Beeper Mode" {
            n198 = Pick Line(multi-line string="OFF\nGD\nNG", line index=w460) -> (output string=w464:string)  [unwired: 1 in]
            n199 = Format Into String(format string=":BIN:BEEP %s;", w464) -> (resulting string=w461:string)  [unwired: 2 in, 1 out]
            n200 = call "Write.vi"("Input String"=w461, "error in (no error)"=w467, "VISA resource name"=w465) -> ("error out"=w466:errorcluster)  [unwired: 7 in, 1 out]
          }
        }
      }
      frame "LowNominal" {
        # "Sets the Lower Limit or Nominal Value depending on the selected BIN Mode."
        n201 = local read "Nominal REF"() -> (w469:refnum<vi>)
        n202 = Unbundle By Name(w472) -> ("Hardware Configuration.Inst."=w471:refnum<visa-resource-name>)
        n203 = property class="DigNum (strict)"(reference=w469) -> ("Label.Text"=w468:string)  [unwired: 1 in, 2 out]
        n204 = local read "Nom New Val"() -> (w473:dbl)
        n205 = property on="Nominal" class="Clust (strict)"() -> ("Caption.Text"=w476:string)  [unwired: 2 in, 2 out]
        n206 = case shown="\"Nominal\"" w476 {
          tunnel: w475 -> [w478 w482 w547]
          tunnel: [w478 w481 w546] -> w474
          tunnel: w468 -> [_ w483 w549]
          tunnel: w473 -> [_ w480 w545]
          tunnel: w471 -> [_ w479 w548]
          frame "False", Default {
          }
          frame "Lower Limit" {
            n207 = case shown="\"BIN 1\"" w483 {
              tunnel: w482 -> [w484 w490 w496 w502 w508 w514 w520 w526 w532 w538 w544]
              tunnel: [w484 w489 w495 w501 w507 w513 w519 w525 w531 w537 w543] -> w481
              tunnel: w480 -> [_ w487 w493 w499 w505 w511 w517 w523 w529 w535 w541]
              tunnel: w479 -> [_ w485 w491 w497 w503 w509 w515 w521 w527 w533 w539]
              frame "False", Default {
              }
              frame "BIN 1" {
                n208 = Format Into String(format string=":BIN:LOW 1,%f;", w487) -> (resulting string=w486:string)  [unwired: 2 in, 1 out]
                n209 = call "Write.vi"("Input String"=w486, "error in (no error)"=w490, "VISA resource name"=w485) -> ("error out"=w489:errorcluster)  [unwired: 7 in, 1 out]
              }
              frame "BIN 2" {
                n210 = Format Into String(format string=":BIN:LOW 2,%f;", w493) -> (resulting string=w492:string)  [unwired: 2 in, 1 out]
                n211 = call "Write.vi"("Input String"=w492, "error in (no error)"=w496, "VISA resource name"=w491) -> ("error out"=w495:errorcluster)  [unwired: 7 in, 1 out]
              }
              frame "BIN 3" {
                n212 = Format Into String(format string=":BIN:LOW 3,%f;", w499) -> (resulting string=w498:string)  [unwired: 2 in, 1 out]
                n213 = call "Write.vi"("Input String"=w498, "error in (no error)"=w502, "VISA resource name"=w497) -> ("error out"=w501:errorcluster)  [unwired: 7 in, 1 out]
              }
              frame "BIN 4" {
                n214 = Format Into String(format string=":BIN:LOW 4,%f;", w505) -> (resulting string=w504:string)  [unwired: 2 in, 1 out]
                n215 = call "Write.vi"("Input String"=w504, "error in (no error)"=w508, "VISA resource name"=w503) -> ("error out"=w507:errorcluster)  [unwired: 7 in, 1 out]
              }
              frame "BIN 5" {
                n216 = Format Into String(format string=":BIN:LOW 5,%f;", w511) -> (resulting string=w510:string)  [unwired: 2 in, 1 out]
                n217 = call "Write.vi"("Input String"=w510, "error in (no error)"=w514, "VISA resource name"=w509) -> ("error out"=w513:errorcluster)  [unwired: 7 in, 1 out]
              }
              frame "BIN 6" {
                n218 = Format Into String(format string=":BIN:LOW 6,%f;", w517) -> (resulting string=w516:string)  [unwired: 2 in, 1 out]
                n219 = call "Write.vi"("Input String"=w516, "error in (no error)"=w520, "VISA resource name"=w515) -> ("error out"=w519:errorcluster)  [unwired: 7 in, 1 out]
              }
              frame "BIN 7" {
                n220 = Format Into String(format string=":BIN:LOW 7,%f;", w523) -> (resulting string=w522:string)  [unwired: 2 in, 1 out]
                n221 = call "Write.vi"("Input String"=w522, "error in (no error)"=w526, "VISA resource name"=w521) -> ("error out"=w525:errorcluster)  [unwired: 7 in, 1 out]
              }
              frame "BIN 8" {
                n222 = Format Into String(format string=":BIN:LOW 8,%f;", w529) -> (resulting string=w528:string)  [unwired: 2 in, 1 out]
                n223 = call "Write.vi"("Input String"=w528, "error in (no error)"=w532, "VISA resource name"=w527) -> ("error out"=w531:errorcluster)  [unwired: 7 in, 1 out]
              }
              frame "BIN 9" {
                n224 = Format Into String(format string=":BIN:LOW 9,%f;", w535) -> (resulting string=w534:string)  [unwired: 2 in, 1 out]
                n225 = call "Write.vi"("Input String"=w534, "error in (no error)"=w538, "VISA resource name"=w533) -> ("error out"=w537:errorcluster)  [unwired: 7 in, 1 out]
              }
              frame "BIN 10" {
                n226 = Format Into String(format string=":BIN:LOW 10,%f;", w541) -> (resulting string=w540:string)  [unwired: 2 in, 1 out]
                n227 = call "Write.vi"("Input String"=w540, "error in (no error)"=w544, "VISA resource name"=w539) -> ("error out"=w543:errorcluster)  [unwired: 7 in, 1 out]
              }
            }
          }
          frame "Nominal" {
            n228 = case shown="\"BIN 1\"" w549 {
              tunnel: w547 -> [w550 w556 w562 w568 w574 w580 w586 w592 w598 w604 w610]
              tunnel: [w550 w555 w561 w567 w573 w579 w585 w591 w597 w603 w609] -> w546
              tunnel: w545 -> [_ w553 w559 w565 w571 w577 w583 w589 w595 w601 w607]
              tunnel: w548 -> [_ w551 w557 w563 w569 w575 w581 w587 w593 w599 w605]
              frame "False", Default {
              }
              frame "BIN 1" {
                n229 = Format Into String(format string=":BIN:REF 1,%f;", w553) -> (resulting string=w552:string)  [unwired: 2 in, 1 out]
                n230 = call "Write.vi"("Input String"=w552, "error in (no error)"=w556, "VISA resource name"=w551) -> ("error out"=w555:errorcluster)  [unwired: 7 in, 1 out]
              }
              frame "BIN 2" {
                n231 = Format Into String(format string=":BIN:REF 2,%f;", w559) -> (resulting string=w558:string)  [unwired: 2 in, 1 out]
                n232 = call "Write.vi"("Input String"=w558, "error in (no error)"=w562, "VISA resource name"=w557) -> ("error out"=w561:errorcluster)  [unwired: 7 in, 1 out]
              }
              frame "BIN 3" {
                n233 = Format Into String(format string=":BIN:REF 3,%f;", w565) -> (resulting string=w564:string)  [unwired: 2 in, 1 out]
                n234 = call "Write.vi"("Input String"=w564, "error in (no error)"=w568, "VISA resource name"=w563) -> ("error out"=w567:errorcluster)  [unwired: 7 in, 1 out]
              }
              frame "BIN 4" {
                n235 = Format Into String(format string=":BIN:REF 4,%f;", w571) -> (resulting string=w570:string)  [unwired: 2 in, 1 out]
                n236 = call "Write.vi"("Input String"=w570, "error in (no error)"=w574, "VISA resource name"=w569) -> ("error out"=w573:errorcluster)  [unwired: 7 in, 1 out]
              }
              frame "BIN 5" {
                n237 = Format Into String(format string=":BIN:REF 5,%f;", w577) -> (resulting string=w576:string)  [unwired: 2 in, 1 out]
                n238 = call "Write.vi"("Input String"=w576, "error in (no error)"=w580, "VISA resource name"=w575) -> ("error out"=w579:errorcluster)  [unwired: 7 in, 1 out]
              }
              frame "BIN 6" {
                n239 = Format Into String(format string=":BIN:REF 6,%f;", w583) -> (resulting string=w582:string)  [unwired: 2 in, 1 out]
                n240 = call "Write.vi"("Input String"=w582, "error in (no error)"=w586, "VISA resource name"=w581) -> ("error out"=w585:errorcluster)  [unwired: 7 in, 1 out]
              }
              frame "BIN 7" {
                n241 = Format Into String(format string=":BIN:REF 7,%f;", w589) -> (resulting string=w588:string)  [unwired: 2 in, 1 out]
                n242 = call "Write.vi"("Input String"=w588, "error in (no error)"=w592, "VISA resource name"=w587) -> ("error out"=w591:errorcluster)  [unwired: 7 in, 1 out]
              }
              frame "BIN 8" {
                n243 = Format Into String(format string=":BIN:REF 8,%f;", w595) -> (resulting string=w594:string)  [unwired: 2 in, 1 out]
                n244 = call "Write.vi"("Input String"=w594, "error in (no error)"=w598, "VISA resource name"=w593) -> ("error out"=w597:errorcluster)  [unwired: 7 in, 1 out]
              }
              frame "BIN 9" {
                n245 = Format Into String(format string=":BIN:REF 9,%f;", w601) -> (resulting string=w600:string)  [unwired: 2 in, 1 out]
                n246 = call "Write.vi"("Input String"=w600, "error in (no error)"=w604, "VISA resource name"=w599) -> ("error out"=w603:errorcluster)  [unwired: 7 in, 1 out]
              }
              frame "BIN 10" {
                n247 = Format Into String(format string=":BIN:REF 10,%f;", w607) -> (resulting string=w606:string)  [unwired: 2 in, 1 out]
                n248 = call "Write.vi"("Input String"=w606, "error in (no error)"=w610, "VISA resource name"=w605) -> ("error out"=w609:errorcluster)  [unwired: 7 in, 1 out]
              }
            }
          }
        }
      }
      frame "UpperTol" {
        # "Sets the Upper Limit or % Tolerance Value depending on the selected BIN Mode."
        n249 = local read "% Tolerance Ref"() -> (w612:refnum<vi>)
        n250 = Unbundle By Name(w616) -> ("Hardware Configuration.Inst."=w615:refnum<visa-resource-name>)
        n251 = property class="DigNum (strict)"(reference=w612) -> ("Label.Text"=w611:string)  [unwired: 1 in, 2 out]
        n252 = local read "Tolerance New Val"() -> (w614:dbl)
        n253 = property on="% Tolerance" class="Clust (strict)"() -> ("Caption.Text"=w617:string)  [unwired: 2 in, 2 out]
        n254 = case shown="\"% Tolerance\"" w617 {
          tunnel: w619 -> [w621 w625 w690]
          tunnel: [w621 w624 w689] -> w618
          tunnel: w611 -> [_ w626 w692]
          tunnel: w614 -> [_ w623 w688]
          tunnel: w615 -> [_ w622 w691]
          frame "False", Default {
          }
          frame "Upper Limit" {
            n255 = case shown="\"BIN 1\"" w626 {
              tunnel: w625 -> [w627 w633 w639 w645 w651 w657 w663 w669 w675 w681 w687]
              tunnel: [w627 w632 w638 w644 w650 w656 w662 w668 w674 w680 w686] -> w624
              tunnel: w623 -> [_ w630 w636 w642 w648 w654 w660 w666 w672 w678 w684]
              tunnel: w622 -> [_ w628 w634 w640 w646 w652 w658 w664 w670 w676 w682]
              frame "False", Default {
              }
              frame "BIN 1" {
                n256 = Format Into String(format string=":BIN:UPP 1,%f;", w630) -> (resulting string=w629:string)  [unwired: 2 in, 1 out]
                n257 = call "Write.vi"("Input String"=w629, "error in (no error)"=w633, "VISA resource name"=w628) -> ("error out"=w632:errorcluster)  [unwired: 7 in, 1 out]
              }
              frame "BIN 2" {
                n258 = Format Into String(format string=":BIN:UPP 2,%f;", w636) -> (resulting string=w635:string)  [unwired: 2 in, 1 out]
                n259 = call "Write.vi"("Input String"=w635, "error in (no error)"=w639, "VISA resource name"=w634) -> ("error out"=w638:errorcluster)  [unwired: 7 in, 1 out]
              }
              frame "BIN 3" {
                n260 = Format Into String(format string=":BIN:UPP 3,%f;", w642) -> (resulting string=w641:string)  [unwired: 2 in, 1 out]
                n261 = call "Write.vi"("Input String"=w641, "error in (no error)"=w645, "VISA resource name"=w640) -> ("error out"=w644:errorcluster)  [unwired: 7 in, 1 out]
              }
              frame "BIN 4" {
                n262 = Format Into String(format string=":BIN:UPP 4,%f;", w648) -> (resulting string=w647:string)  [unwired: 2 in, 1 out]
                n263 = call "Write.vi"("Input String"=w647, "error in (no error)"=w651, "VISA resource name"=w646) -> ("error out"=w650:errorcluster)  [unwired: 7 in, 1 out]
              }
              frame "BIN 5" {
                n264 = Format Into String(format string=":BIN:UPP 5,%f;", w654) -> (resulting string=w653:string)  [unwired: 2 in, 1 out]
                n265 = call "Write.vi"("Input String"=w653, "error in (no error)"=w657, "VISA resource name"=w652) -> ("error out"=w656:errorcluster)  [unwired: 7 in, 1 out]
              }
              frame "BIN 6" {
                n266 = Format Into String(format string=":BIN:UPP 6,%f;", w660) -> (resulting string=w659:string)  [unwired: 2 in, 1 out]
                n267 = call "Write.vi"("Input String"=w659, "error in (no error)"=w663, "VISA resource name"=w658) -> ("error out"=w662:errorcluster)  [unwired: 7 in, 1 out]
              }
              frame "BIN 7" {
                n268 = Format Into String(format string=":BIN:UPP 7,%f;", w666) -> (resulting string=w665:string)  [unwired: 2 in, 1 out]
                n269 = call "Write.vi"("Input String"=w665, "error in (no error)"=w669, "VISA resource name"=w664) -> ("error out"=w668:errorcluster)  [unwired: 7 in, 1 out]
              }
              frame "BIN 8" {
                n270 = Format Into String(format string=":BIN:UPP 8,%f;", w672) -> (resulting string=w671:string)  [unwired: 2 in, 1 out]
                n271 = call "Write.vi"("Input String"=w671, "error in (no error)"=w675, "VISA resource name"=w670) -> ("error out"=w674:errorcluster)  [unwired: 7 in, 1 out]
              }
              frame "BIN 9" {
                n272 = Format Into String(format string=":BIN:UPP 9,%f;", w678) -> (resulting string=w677:string)  [unwired: 2 in, 1 out]
                n273 = call "Write.vi"("Input String"=w677, "error in (no error)"=w681, "VISA resource name"=w676) -> ("error out"=w680:errorcluster)  [unwired: 7 in, 1 out]
              }
              frame "BIN 10" {
                n274 = Format Into String(format string=":BIN:UPP 10,%f;", w684) -> (resulting string=w683:string)  [unwired: 2 in, 1 out]
                n275 = call "Write.vi"("Input String"=w683, "error in (no error)"=w687, "VISA resource name"=w682) -> ("error out"=w686:errorcluster)  [unwired: 7 in, 1 out]
              }
            }
          }
          frame "% Tolerance" {
            n276 = case shown="\"BIN 1\"" w692 {
              tunnel: w690 -> [w693 w699 w705 w711 w717 w723 w729 w735 w741 w747 w753]
              tunnel: [w693 w698 w704 w710 w716 w722 w728 w734 w740 w746 w752] -> w689
              tunnel: w688 -> [_ w696 w702 w708 w714 w720 w726 w732 w738 w744 w750]
              tunnel: w691 -> [_ w694 w700 w706 w712 w718 w724 w730 w736 w742 w748]
              frame "False", Default {
              }
              frame "BIN 1" {
                n277 = Format Into String(format string=":BIN:PERC 1,%f;", w696) -> (resulting string=w695:string)  [unwired: 2 in, 1 out]
                n278 = call "Write.vi"("Input String"=w695, "error in (no error)"=w699, "VISA resource name"=w694) -> ("error out"=w698:errorcluster)  [unwired: 7 in, 1 out]
              }
              frame "BIN 2" {
                n279 = Format Into String(format string=":BIN:PERC 2,%f;", w702) -> (resulting string=w701:string)  [unwired: 2 in, 1 out]
                n280 = call "Write.vi"("Input String"=w701, "error in (no error)"=w705, "VISA resource name"=w700) -> ("error out"=w704:errorcluster)  [unwired: 7 in, 1 out]
              }
              frame "BIN 3" {
                n281 = Format Into String(format string=":BIN:PERC 3,%f;", w708) -> (resulting string=w707:string)  [unwired: 2 in, 1 out]
                n282 = call "Write.vi"("Input String"=w707, "error in (no error)"=w711, "VISA resource name"=w706) -> ("error out"=w710:errorcluster)  [unwired: 7 in, 1 out]
              }
              frame "BIN 4" {
                n283 = Format Into String(format string=":BIN:PERC 4,%f;", w714) -> (resulting string=w713:string)  [unwired: 2 in, 1 out]
                n284 = call "Write.vi"("Input String"=w713, "error in (no error)"=w717, "VISA resource name"=w712) -> ("error out"=w716:errorcluster)  [unwired: 7 in, 1 out]
              }
              frame "BIN 5" {
                n285 = Format Into String(format string=":BIN:PERC 5,%f;", w720) -> (resulting string=w719:string)  [unwired: 2 in, 1 out]
                n286 = call "Write.vi"("Input String"=w719, "error in (no error)"=w723, "VISA resource name"=w718) -> ("error out"=w722:errorcluster)  [unwired: 7 in, 1 out]
              }
              frame "BIN 6" {
                n287 = Format Into String(format string=":BIN:PERC 6,%f;", w726) -> (resulting string=w725:string)  [unwired: 2 in, 1 out]
                n288 = call "Write.vi"("Input String"=w725, "error in (no error)"=w729, "VISA resource name"=w724) -> ("error out"=w728:errorcluster)  [unwired: 7 in, 1 out]
              }
              frame "BIN 7" {
                n289 = Format Into String(format string=":BIN:PERC 7,%f;", w732) -> (resulting string=w731:string)  [unwired: 2 in, 1 out]
                n290 = call "Write.vi"("Input String"=w731, "error in (no error)"=w735, "VISA resource name"=w730) -> ("error out"=w734:errorcluster)  [unwired: 7 in, 1 out]
              }
              frame "BIN 8" {
                n291 = Format Into String(format string=":BIN:PERC 8,%f;", w738) -> (resulting string=w737:string)  [unwired: 2 in, 1 out]
                n292 = call "Write.vi"("Input String"=w737, "error in (no error)"=w741, "VISA resource name"=w736) -> ("error out"=w740:errorcluster)  [unwired: 7 in, 1 out]
              }
              frame "BIN 9" {
                n293 = Format Into String(format string=":BIN:PERC 9,%f;", w744) -> (resulting string=w743:string)  [unwired: 2 in, 1 out]
                n294 = call "Write.vi"("Input String"=w743, "error in (no error)"=w747, "VISA resource name"=w742) -> ("error out"=w746:errorcluster)  [unwired: 7 in, 1 out]
              }
              frame "BIN 10" {
                n295 = Format Into String(format string=":BIN:PERC 10,%f;", w750) -> (resulting string=w749:string)  [unwired: 2 in, 1 out]
                n296 = call "Write.vi"("Input String"=w749, "error in (no error)"=w753, "VISA resource name"=w748) -> ("error out"=w752:errorcluster)  [unwired: 7 in, 1 out]
              }
            }
          }
        }
      }
      frame "BIN State" {
        # "Enable/disable BINs"
        n297 = local read "BIN NO. Ref"() -> (w755:refnum<vi>)
        n298 = property class="Bool (strict)"(reference=w755) -> ("Label.Text"=w754:string)  [unwired: 1 in, 2 out]
        n299 = local read "BIN No.State"() -> (w764:bool)
        n300 = case shown="\"BIN 2\"" w754 {
          tunnel: w764 -> [_ w770 w774 w778 w782 w786 w790 w794 w798 w802 w806]
          tunnel: [0 w769 w773 w777 w781 w785 w789 w793 w797 w801 w805] -> w763
          frame "False", Default {
          }
          frame "BIN 1" {
            n301 = Select(t=1, s=w770, f=-1) -> (s? t:f=w769:i32)
          }
          frame "BIN 2" {
            n302 = Select(t=2, s=w774, f=-2) -> (s? t:f=w773:i32)
          }
          frame "BIN 3" {
            n303 = Select(t=4, s=w778, f=-4) -> (s? t:f=w777:i32)
          }
          frame "BIN 4" {
            n304 = Select(t=8, s=w782, f=-8) -> (s? t:f=w781:i32)
          }
          frame "BIN 5" {
            n305 = Select(t=16, s=w786, f=-16) -> (s? t:f=w785:i32)
          }
          frame "BIN 6" {
            n306 = Select(t=32, s=w790, f=-32) -> (s? t:f=w789:i32)
          }
          frame "BIN 7" {
            n307 = Select(t=64, s=w794, f=-64) -> (s? t:f=w793:i32)
          }
          frame "BIN 8" {
            n308 = Select(t=128, s=w798, f=-128) -> (s? t:f=w797:i32)
          }
          frame "BIN 9" {
            n309 = Select(t=256, s=w802, f=-256) -> (s? t:f=w801:i32)
          }
          frame "BIN 10" {
            n310 = Select(t=512, s=w806, f=-512) -> (s? t:f=w805:i32)
          }
        }
        n311 = local read "BIN State Value"() -> (w760:i32)
        n312 = Unbundle By Name(w757) -> ("Hardware Configuration.Inst."=w756:refnum<visa-resource-name>)
        n313 = Add(x=w763, y=w760) -> (x+y=w762:i32)
        n314 = Format Into String(format string=":BIN:ENAB %d;", w762) -> (resulting string=w758:string)  [unwired: 2 in, 1 out]
        n315 = local write "BIN State Value"(w762) -> ()
        n316 = call "Write.vi"("Input String"=w758, "error in (no error)"=w761, "VISA resource name"=w756) -> ("error out"=w765:errorcluster)  [unwired: 7 in, 1 out]
      }
      frame "Configure Comparator" {
        # "Congfigure the comparator settings.(State, Mode, Beeper, Upper, Lower)"
        n317 = local read "COMP Ref"() -> (w820:refnum<vi>)
        n318 = Unbundle By Name(w812) -> ("Hardware Configuration.Inst."=w815:refnum<visa-resource-name>)
        n319 = property class="Ctl"(reference=w820) -> ("Label.Text"=w819:string)  [unwired: 1 in, 2 out]
        n320 = local read "Comparator Mode"() -> (w814:u16)
        n321 = case shown="\"COMP State\"" w819 {
          tunnel: "COMP State" -> [_ w824 _ _ _ _]
          tunnel: w817 -> [w822 w835 w856 w864 w881 w899]
          tunnel: [w822 w840 w855 w862 w880 w898] -> w816
          tunnel: w815 -> [_ w839 w854 w863 w879 w897]
          tunnel: w814 -> [_ _ w849 w865 w882 _]
          tunnel: w812 -> [w821 w837 w845 w861 w878 w895]
          tunnel: [w821 w836 w845 w861 w878 w895] -> w811
          tunnel: w810 -> [_ w832 _ _ _ _]
          tunnel: w809 -> [_ w831 _ _ _ _]
          frame "False", Default {
          }
          frame "COMP State" {
            n322 = Not(x=w824) -> (.not. x?=w823:bool)
            n323 = call-poly "Enqueue Message.vi"("error in (no error)"=w835, "Message"="Broadcast settings", "Message Queue"=w832) -> ("error out"=w834:errorcluster)  [unwired: 7 in, 1 out]
            n324 = Bundle By Name(cluster=w837, "Hardware Configuration.COMP State"=w824) -> (w836:T8)
            n325 = Unbundle By Name(w831) -> ("COMP Trig"=w830:refnum<vi>, "COMP Mode"=w829:refnum<vi>, "COMP Beeper"=w828:refnum<vi>, "COMP  Tol"=w827:refnum<vi>, "COMP  Nom"=w826:refnum<vi>)
            n326 = Select(t=1, s=w824, f=0) -> (s? t:f=w838:i32)
            n327 = Format Into String(format string="COMP %d;::COMP:COUN %d;", w838, w838) -> (resulting string=w841:string)  [unwired: 2 in, 1 out]
            n328 = Build Array(w830, w829, w828, w827, w826) -> (w825:refnum<vi>[])
            n329 = call "Write.vi"("Input String"=w841, "error in (no error)"=w834, "VISA resource name"=w839) -> ("error out"=w840:errorcluster)  [unwired: 7 in, 1 out]
            n330 = call "Set Enable State on Multiple Controls.vi"("Enable?"=w823, "Controls"=w825) -> ()  [unwired: 10 in]
          }
          frame "Comparator Mode" {
            n331 = Equal To 0?(x=w849) -> (x = 0?=w848:bool)
            n332 = Pick Line(multi-line string="PTOL\nATOL", line index=w849) -> (output string=w858:string)  [unwired: 1 in]
            n333 = Format Into String(format string=":COMP:MODE %s;" ("true string"), w858) -> (resulting string=w857:string)  [unwired: 2 in, 1 out]
            n334 = call "Write.vi"("Input String"=w857, "error in (no error)"=w856, "VISA resource name"=w854) -> ("error out"=w855:errorcluster)  [unwired: 7 in, 1 out]
            n335 = Select(t="Nominal", s=w848, f="Upper Limit") -> (s? t:f=w846:string)
            n336 = Select(t="% Tolerance", s=w848, f="Lower Limit") -> (s? t:f=w847:string)
            n337 = property on="Comparator Upper" class="DigNum (strict)"("Caption.Text"=w846) -> ()  [unwired: 2 in, 2 out]
            n338 = property on="Comparator Lower" class="DigNum (strict)"("Caption.Text"=w847) -> ()  [unwired: 2 in, 2 out]
          }
          frame "Comparator Upper" {
            n339 = case shown="1" w865 {
              tunnel: w864 -> [w871 w874]
              tunnel: w863 -> [w870 w873]
              tunnel: [w869 w872] -> w862
              frame 0, Default {
                n340 = local read "Comparator Upper"() -> (w868:dbl)
                n341 = Format Into String(format string=":COMP:REF %f;", w868) -> (resulting string=w866:string)  [unwired: 2 in, 1 out]
                n342 = call "Write.vi"("Input String"=w866, "error in (no error)"=w871, "VISA resource name"=w870) -> ("error out"=w869:errorcluster)  [unwired: 7 in, 1 out]
              }
              frame 1 {
                n343 = local read "Comparator Upper"() -> (w876:dbl)
                n344 = Format Into String(format string=":COMP:UPP %f;", w876) -> (resulting string=w875:string)  [unwired: 2 in, 1 out]
                n345 = call "Write.vi"("Input String"=w875, "error in (no error)"=w874, "VISA resource name"=w873) -> ("error out"=w872:errorcluster)  [unwired: 7 in, 1 out]
              }
            }
          }
          frame "Comparator Lower" {
            n346 = case shown="0, Default" w882 {
              tunnel: w881 -> [w887 w894]
              tunnel: [w885 w893] -> w880
              tunnel: w879 -> [w886 w892]
              frame 0, Default {
                n347 = local read "Comparator Lower"() -> (w883:dbl)
                n348 = Format Into String(format string=":COMP:PERC %f;", w883) -> (resulting string=w884:string)  [unwired: 2 in, 1 out]
                n349 = call "Write.vi"("Input String"=w884, "error in (no error)"=w887, "VISA resource name"=w886) -> ("error out"=w885:errorcluster)  [unwired: 7 in, 1 out]
              }
              frame 1 {
                n350 = local read "Comparator Lower"() -> (w889:dbl)
                n351 = Format Into String(format string=":COMP:LOW %f;", w889) -> (resulting string=w890:string)  [unwired: 2 in, 1 out]
                n352 = call "Write.vi"("Input String"=w890, "error in (no error)"=w894, "VISA resource name"=w892) -> ("error out"=w893:errorcluster)  [unwired: 7 in, 1 out]
              }
            }
          }
          frame "Comparator Clear" {
            n353 = call "Write.vi"("Input String"=":COMP:COUN:CLEAR;" ("format string"), "error in (no error)"=w899, "VISA resource name"=w897) -> ("error out"=w898:errorcluster)  [unwired: 7 in, 1 out]
          }
        }
      }
      frame "Update Status" {
        # "Update Status - Convert the message data to a string to display in the Status indicator."
        n354 = Variant To Data(error in=w907, type="", Variant=w906) -> (data=→"Status":string, error out=w900:errorcluster)
      }
      frame "Start Logging" {
        # "Message Acquisition and Logging loops to start."
        # "Enable: Stop\nDisable: Start, Exit, Settings"
        # "Start - Enable/Disable buttons appropriately for data logging that has started, and update status display."
        n355 = Unbundle By Name(w921) -> ("Stop Ref"=w916:refnum<vi>, "Start Ref"=w915:refnum<vi>, "Exit Ref"=w914:refnum<vi>, "Settings Ref"=w913:refnum<vi>)
        n356 = call-poly "Enqueue Message.vi"("error in (no error)"=w925, "Message Data"="Acquiring and Logging..." ("Acquiring and Logging..."), "Message"="Update Status", "Message Queue"=w926) -> ("error out"=w912:errorcluster)  [unwired: 6 in, 1 out]
        n357 = Build Array(w915, w914, w913) -> (w919:refnum<vi>[])
        n358 = Build Array(w916) -> (w918:refnum<vi>[])
        n359 = call "Set Enable State on Multiple Controls.vi"("Enable?"=TRUE, "Controls"=w918) -> ()  [unwired: 10 in]
        n360 = call "Set Enable State on Multiple Controls.vi"("Enable?"=FALSE, "Controls"=w919) -> ()  [unwired: 10 in]
        n361 = call-poly "Enqueue Message.vi"("error in (no error)"=w912, "Message"="Start", "Message Queue"=w910) -> ("error out"=w909:errorcluster)  [unwired: 7 in, 1 out]
      }
      frame "Start Acquire" {
        # "Message Acquisition and Logging loops to start."
        # "Start - Enable/Disable buttons appropriately for data acquisition that has started, and update status display."
        n362 = call-poly "Enqueue Message.vi"("error in (no error)"=w936, "Message Data"="Acquiring ..." ("Acquiring and Logging..."), "Message"="Update Status", "Message Queue"=w937) -> ("error out"=w931:errorcluster)  [unwired: 6 in, 1 out]
        n363 = call-poly "Enqueue Message.vi"("error in (no error)"=w931, "Message"="Acquire", "Message Queue"=w928) -> ("error out"=w929:errorcluster)  [unwired: 7 in, 1 out]
      }
      frame "Stop" {
        # "Message Acquisition and Logging loops to stop"
        # "Enable: Start, Exit, Settings\nDisable: Stop"
        # "Stop - Enable/Disable buttons appropriately for an acquisition that has stopped, and update status display."
        n364 = Unbundle By Name(w951) -> ("Stop Ref"=w946:refnum<vi>, "Start Ref"=w945:refnum<vi>, "Exit Ref"=w944:refnum<vi>, "Settings Ref"=w943:refnum<vi>)
        n365 = Build Array(w945, w944, w943) -> (w949:refnum<vi>[])
        n366 = Build Array(w946) -> (w948:refnum<vi>[])
        n367 = call "Set Enable State on Multiple Controls.vi"("Enable?"=FALSE, "Controls"=w948) -> ()  [unwired: 10 in]
        n368 = call "Set Enable State on Multiple Controls.vi"("Enable?"=TRUE, "Controls"=w949) -> ()  [unwired: 10 in]
        n369 = call-poly "Enqueue Message.vi"("error in (no error)"=w953, "Message"="Stop", "Message Queue"=w941) -> ("error out"=w940:errorcluster)  [unwired: 7 in, 1 out]
        n370 = case shown="Default" w938 {
          selector: w938 -> [w954 _]
          tunnel: [w954 UI_State."Waiting for Stop" ("UI State")] -> w939
          frame "Waiting for Exit" {
          }
          frame Default {
          }
        }
      }
      frame "Acquisition Stopped" {
        # "Logic for determining what action to take when the acquisition has stopped."
        n371 = case shown="\"Waiting for Stop\", \"Waiting for Stop (Acq Stopped)\"" w960 {
          selector: w960 -> [w964 _ _ _ _]
          tunnel: w959 -> [w963 w966 w968 w974 w980]
          tunnel: w958 -> [_ _ _ w972 w977]
          tunnel: [w964 UI_State."Waiting for Exit (Acq Stopped)" ("UI State") UI_State."Waiting for Stop (Acq Stopped)" ("UI State") UI_State."Idle" ("UI State") UI_State."Idle" ("UI State")] -> w957
          tunnel: [w963 w966 w968 w973 w978] -> w956
          frame Default {
          }
          frame "Waiting for Exit", "Waiting for Exit (Acq Stopped)" {
          }
          frame "Waiting for Stop", "Waiting for Stop (Acq Stopped)" {
          }
          frame "Waiting for Exit (Log Stopped)" {
            # "If we are waiting to exit, and the logging has already stopped, then the \"Acquisition Stopped\" message indicates that it is time to exit."
            n372 = call-poly "Enqueue Message.vi"("Priority Message? (F)"=TRUE, "error in (no error)"=w974, "Message"="Exit", "Message Queue"=w972) -> ("error out"=w973:errorcluster)  [unwired: 6 in, 1 out]
          }
          frame "Waiting for Stop (Log Stopped)" {
            # "If we are waiting to stop, and the logging has already stopped, then the \"Acquisition Stopped\" message indicates that it is time to stop."
            n373 = call-poly "Enqueue Message.vi"("error in (no error)"=w980, "Message Data"="Ready..." ("Ready..."), "Message"="Update Status", "Message Queue"=w977) -> ("error out"=w978:errorcluster)  [unwired: 6 in, 1 out]
          }
        }
      }
      frame "Logging Stopped" {
        # "Enable: Start, Exit, Settings\nDisable: Stop"
        # "Logic for determining what action to take when the logging has stopped."
        n374 = Unbundle By Name(w981) -> ("Stop Ref"=w985:refnum<vi>, "Start Ref"=w984:refnum<vi>, "Exit Ref"=w983:refnum<vi>, "Settings Ref"=w982:refnum<vi>)
        n375 = case shown="\"Waiting for Exit (Acq Stopped)\"" w994 {
          selector: w994 -> [w997 _ _ _ _]
          tunnel: w993 -> [w996 w999 w1001 w1007 w1010]
          tunnel: w992 -> [_ _ _ w1005 w1009]
          tunnel: [w997 UI_State."Waiting for Exit (Log Stopped)" ("UI State") UI_State."Waiting for Stop (Log Stopped)" ("UI State") UI_State."Idle" ("UI State") UI_State."Idle" ("UI State")] -> w991
          tunnel: [w996 w999 w1001 w1006 w1008] -> w990
          frame Default {
          }
          frame "Waiting for Exit", "Waiting for Exit (Log Stopped)" {
          }
          frame "Waiting for Stop", "Waiting for Stop (Log Stopped)" {
          }
          frame "Waiting for Exit (Acq Stopped)" {
            # "If we are waiting to exit, and the acquisition has already stopped, then the \"Logging Stopped\" message indicates that it is time to exit."
            n376 = call-poly "Enqueue Message.vi"("Priority Message? (F)"=TRUE, "error in (no error)"=w1007, "Message"="Exit", "Message Queue"=w1005) -> ("error out"=w1006:errorcluster)  [unwired: 6 in, 1 out]
          }
          frame "Waiting for Stop (Acq Stopped)" {
            # "If we are waiting to stop, and the acquisition has already stopped, then the \"Logging Stopped\" message indicates that it is time to stop."
            n377 = call-poly "Enqueue Message.vi"("error in (no error)"=w1010, "Message Data"="Ready..." ("Ready..."), "Message"="Update Status", "Message Queue"=w1009) -> ("error out"=w1008:errorcluster)  [unwired: 6 in, 1 out]
          }
        }
        n378 = Build Array(w984, w983, w982) -> (w988:refnum<vi>[])
        n379 = Build Array(w985) -> (w987:refnum<vi>[])
        n380 = call "Set Enable State on Multiple Controls.vi"("Enable?"=FALSE, "Controls"=w987) -> ()  [unwired: 10 in]
        n381 = call "Set Enable State on Multiple Controls.vi"("Enable?"=TRUE, "Controls"=w988) -> ()  [unwired: 10 in]
      }
      frame "Broadcast settings" {
        w1024 = "Update Settings" ("Message")
        # "Broadcast settings - Send the 'Update Settings' message to the Logging and Acquisition message loops."
        n382 = Unbundle By Name(w1025) -> ("Hardware Configuration"=w1018:T9, "Logging Configuration"=w1019:T10)
        n383 = call-poly "Enqueue Message.vi"("Message Data"=w1019, "Message"=w1024, "Message Queue"=w1020) -> ("error out"=w1026:errorcluster)  [unwired: 7 in, 1 out]
        n384 = Unbundle By Name(w1018) -> ("Trigger Source"=w1017:u16)
        n385 = call-poly "Enqueue Message.vi"("error in (no error)"=w1026, "Message Data"=w1018, "Message"=w1024, "Message Queue"=w1021) -> ("error out"=w1016:errorcluster)  [unwired: 6 in, 1 out]
        n386 = case shown="3" w1017 {
          tunnel: [w1027 w1028 w1029 w1030] -> w1015
          tunnel: w1016 -> [w1027 w1028 w1029 w1034]
          tunnel: w1014 -> [_ _ _ w1033]
          frame 0, Default {
          }
          frame 1 {
          }
          frame 2 {
          }
          frame 3 {
            n387 = call-poly "Enqueue Message.vi"("error in (no error)"=w1034, "Message Data"="Waiting for trigger ..." ("Acquiring and Logging..."), "Message"="Update Status", "Message Queue"=w1033) -> ("error out"=w1030:errorcluster)  [unwired: 6 in, 1 out]
          }
        }
      }
      frame "Launch Settings Dialog" {
        # "Launch Settings Dialog - Launch the Settings Dialog when the user clicks the 'Settings' button."
        n388 = call-by-ref "?"("error in (no error)"=w1042, "Settings in"=w1043) -> ("error out"=w1038:errorcluster, "Cancelled?"=w1041:bool, "Settings out"=w1039:T8)  [unwired: 8 in, 3 out]
        n389 = case shown="False" w1041 {
          tunnel: w1040 -> [w1047 _]
          tunnel: w1038 -> [w1046 w1048]
          tunnel: [w1045 w1048] -> w1035
          frame False {
            n390 = call-poly "Enqueue Message.vi"("error in (no error)"=w1046, "Message"="Broadcast Settings", "Message Queue"=w1047) -> ("error out"=w1045:errorcluster)  [unwired: 7 in, 1 out]
          }
          frame True {
          }
        }
      }
      frame "Error" {
        # "Error - Display an error dialog. This message is sent by the \"Error Handler\" VIs at the end of other loops in this application."
        n391 = Variant To Data(error in=w1049, type=errorcluster {"status"=FALSE, "code"=0, "source"=""} ("error constant"), Variant=w1052) -> (data=w1050:errorcluster, error out=w1053:errorcluster)
        n392 = call <vilib>:"Simple Error Handler.vi"("error in (no error)"=w1050) -> ()  [unwired: 4 in, 5 out]
      }
      frame "Disconnect" {
        w1057 = T12."Disabled and Grayed Out" ("Disabled")
        w1068 = "stop" ("Message")
        # "Stops data acquisition and logging if loggin is enabled. The session is closed in the acquistion VI."
        n393 = property on="Connect" class="Bool (strict)"("DisabledEnum"=T12."Enabled" ("Disabled")) -> ()  [unwired: 2 in, 2 out]
        n394 = property on="Connect" class="Bool (strict)"() -> ("Value"=w1058:bool)  [unwired: 2 in, 2 out]
        n395 = call-poly "Enqueue Message.vi"("Priority Message? (F)"=TRUE, "error in (no error)"=w1066, "Message"=w1068, "Message Queue"=w1064) -> ("error out"=w1069:errorcluster)  [unwired: 6 in, 1 out]
        n396 = Flush Queue(queue=w1064, error in (no error)=w1066) -> (error out=w1070:errorcluster)  [unwired: 2 out]
        n397 = case shown="True" w1058 {
          tunnel: w1068 -> [_ w1080]
          tunnel: w1069 -> [w1073 w1079]
          tunnel: w1070 -> [w1074 w1078]
          tunnel: [w1074 w1077] -> w1061
          tunnel: [w1073 w1076] -> w1062
          tunnel: w1065 -> [_ w1075]
          frame False {
          }
          frame True {
            n398 = call-poly "Enqueue Message.vi"("error in (no error)"=w1079, "Message"=w1080, "Message Queue"=w1075) -> ("error out"=w1076:errorcluster)  [unwired: 7 in, 1 out]
            n399 = Flush Queue(queue=w1075, error in (no error)=w1078) -> (error out=w1077:errorcluster)  [unwired: 2 out]
          }
        }
        n400 = Merge Errors(w1062, w1061) -> (w1063:errorcluster)
        n401 = property on="Meas Tab" class="TabCtl (strict)"("DisabledEnum"=w1057) -> ()  [unwired: 2 in, 2 out]
        n402 = property on="Tab Control" class="TabCtl (strict)"("DisabledEnum"=w1057) -> ()  [unwired: 2 in, 2 out]
        n403 = property on="Start" class="Bool"("DisabledEnum"=w1057) -> ()  [unwired: 2 in, 2 out]
      }
      frame "Confirm Quit" {
        # "Confirm Quit - Message that can confirm whether or not the user wants to exit the application."
        n404 = case shown="\"Acquiring and Logging\"" w1085 {
          tunnel: w1084 -> [w1093 w1097]
          tunnel: w1083 -> [w1092 w1096]
          tunnel: [w1091 w1095] -> w1082
          tunnel: [UI_State."Idle" ("UI State") w1094] -> w1081
          frame Default {
            # "If 'Confirm Quit' comes in while the system is idle, there is no need for a confirmation message."
            n405 = call-poly "Enqueue Message.vi"("Priority Message? (F)"=TRUE, "error in (no error)"=w1092, "Message"="Exit", "Message Queue"=w1093) -> ("error out"=w1091:errorcluster)  [unwired: 6 in, 1 out]
          }
          frame "Acquiring and Logging" {
            n406 = Two Button Dialog(message="Are you sure you want to quit while the acquisition is running?" ("Confirm Quit Message"), 1:"No" ("No"), 2:"Yes" ("Yes")) -> (T button?=w1098:bool)
            n407 = case shown="True" w1098 {
              tunnel: w1097 -> [_ w1107]
              tunnel: w1096 -> [w1103 w1108]
              tunnel: [w1103 w1106] -> w1095
              tunnel: [UI_State."Acquiring and Logging" ("UI State") UI_State."Waiting for Exit" ("UI State")] -> w1094
              frame False {
                # "User did not want to quit."
              }
              frame True {
                n408 = call-poly "Enqueue Message.vi"("error in (no error)"=w1108, "Message"="Stop", "Message Queue"=w1107) -> ("error out"=w1106:errorcluster)  [unwired: 7 in, 1 out]
              }
            }
          }
        }
      }
      frame "Exit" {
        w1115 = TRUE ("Priority Message? (F)")
        w1116 = "Exit" ("Message")
        # "Popup an error dialog if 'Exit' was called as a result of an error."
        # "Stop the VI"
        # "Exit - Send Exit messages to the Acquisition and Logging loops, and fire the user event to stop the Event Handling Loop."
        n409 = Variant To Data(type=errorcluster {"status"=FALSE, "code"=0, "source"=""} ("error constant"), Variant=w1111) -> (data=w1110:errorcluster)  [unwired: 1 in, 1 out]
        n410 = call <vilib>:"Simple Error Handler.vi"("error in (no error)"=w1110) -> ()  [unwired: 4 in, 5 out]
        n411 = call-poly "Enqueue Message.vi"("Priority Message? (F)"=w1115, "error in (no error)"=w1113, "Message"=w1116, "Message Queue"=w1120) -> ("error out"=w1117:errorcluster)  [unwired: 6 in, 1 out]
        n412 = call-poly "Enqueue Message.vi"("Priority Message? (F)"=w1115, "error in (no error)"=w1117, "Message"=w1116, "Message Queue"=w1119) -> ("error out"=w1114:errorcluster)  [unwired: 6 in, 1 out]
        n413 = property on="Connect" class="Bool (strict)"("DisabledEnum"=T12."Enabled" ("Disabled")) -> ()  [unwired: 2 in, 2 out]
        n414 = call "Fire User Event - Stop.vi"("error in (no error)"=w1114, "User Event - Stop"=w1124) -> ("error out"=w1123:errorcluster)  [unwired: 9 in]
      }
      frame "---Copy This Frame---" {
        # "Duplicate this frame when creating new messages.  Change this comment in the duplicated frame to describe this message."
      }
      frame Default {
        # "'Default' case only runs if there is a message that isn't defined in any of the other cases.  Output a programming error."
        n415 = xnode "Error Ring"("parameter 0"=w1131) -> ("error out"=w1130:errorcluster)
      }
    }
    n416 = call "Error Handler - Message Handling Loop.vi"("error in (no error)"=w40, "Message Queue"=w39) -> ("dup error in"=w41:errorcluster)  [unwired: 8 in, 1 out]
  }
  n417 = while {
    tunnel: w17 -> [w1147]
    tunnel: [w1144] -> w35
    shift-right: [w1146] -> w28
    shift-left: w22 -> [w1148]
    stop <- w1145 stop-if-true
    # "Event Handling Loop"
    n418 = event shown="[13] \"Disconnect\": Value Change" {
      selector: w1148 -> [_ _ _ _ _ _ _ _ _ _ _ _ _ _ _ _ _ _]
      dyn-events: [_ _ _ _ _ _ _ _ _ _ _ _ _ _ _ _ _ _] -> w1146
      timeout: _ -> [_ _ _ _ _ _ _ _ _ _ _ _ _ _ _ _ _ _]
      tunnel: [_ _ _ _ _ _ _ _ _ _ _ _ _ _ _ _ _ TRUE ("Discard?")] -> w1145
      tunnel: w1147 -> [w1152 w1156 w1160 w1163 w1168 w1171 w1175 w1179 w1184 w1189 w1193 w1197 w1201 w1205 w1209 w1212 w1214 w1218]
      tunnel: [w1150 _ _ _ _ _ _ _ _ _ _ _ w1200 _ w1207 _ w1217 _] -> w1143
      tunnel: [w1149 w1155 w1159 w1162 w1167 w1170 w1174 w1178 w1183 w1188 w1192 w1196 w1199 w1204 w1208 w1212 w1213 w1218] -> w1142
      event "Start": Value Change {
        n419 = event-data() -> ()  [unwired: 1 in, 1 out]
        n420 = call-poly "Enqueue Message.vi"("Message"="Start Logging", "Message Queue"=w1152) -> ("error out"=w1150:errorcluster, "dup Message Queue"=w1149:refnum<queue>)  [unwired: 8 in]
      }
      event "Connect": Value Change {
        n421 = event-data() -> ()  [unwired: 1 in, 1 out]
        n422 = invoke class="VI" method="Default Vals.Reinit All"() -> ()  [unwired: 3 in, 3 out]
        n423 = call-poly "Enqueue Message.vi"("Message"="Init INST.", "Message Queue"=w1156) -> ("dup Message Queue"=w1155:refnum<queue>)  [unwired: 8 in, 1 out]
        n424 = property on="Connect" class="Bool (strict)"("DisabledEnum"=T12."Disabled and Grayed Out" ("Disabled")) -> ()  [unwired: 2 in, 2 out]
      }
      event "Tab Control", "Meas Tab": Value Change {
        n425 = event-data() -> ("CtlRef"=→"Tab Ref":refnum<vi>)  [unwired: 1 in, 5 out]
        n426 = call-poly "Enqueue Message.vi"("Message"="Display Page", "Message Queue"=w1160) -> ("dup Message Queue"=w1159:refnum<queue>)  [unwired: 8 in, 1 out]
      }
      event "Average Readings", "Auto Range", "Manual Range", "Aperture", "Function": Value Change {
        n427 = event-data() -> ("CtlRef"=→"Meas Ctl":refnum<vi>)  [unwired: 1 in, 1 out]
        n428 = call-poly "Enqueue Message.vi"("Message"="Configure Meas", "Message Queue"=w1163) -> ("dup Message Queue"=w1162:refnum<queue>)  [unwired: 8 in, 1 out]
      }
      event "Trigger Source", "Auto Delay", "Manual Trigger Delay", "Trigger 2": Value Change {
        n429 = event-data() -> ("CtlRef"=→"Trigger Ref":refnum<vi>)  [unwired: 1 in, 5 out]
        n430 = call-poly "Enqueue Message.vi"("Message"="Configure Trigger", "Message Queue"=w1168) -> ("dup Message Queue"=w1167:refnum<queue>)  [unwired: 8 in, 1 out]
      }
      event "State", "Statistics Mode", "Nominal", "Deviation", "Statistics Clear", "Trigger": Value Change {
        n431 = event-data() -> ("CtlRef"=→"Stat Ref":refnum<vi>)  [unwired: 1 in, 5 out]
        n432 = call-poly "Enqueue Message.vi"("Message"="Statistics Configuration", "Message Queue"=w1171) -> ("dup Message Queue"=w1170:refnum<queue>)  [unwired: 8 in, 1 out]
      }
      event "BIN State", "Beeper Mode", "BIN Mode": Value Change {
        n433 = event-data() -> ("CtlRef"=→"BIN Event Ref":refnum<vi>)  [unwired: 1 in, 5 out]
        n434 = call-poly "Enqueue Message.vi"("Message"="BIN Configuration", "Message Queue"=w1175) -> ("dup Message Queue"=w1174:refnum<queue>)  [unwired: 8 in, 1 out]
      }
      event "Nominal.BIN 1", "Nominal.BIN 2", "Nominal.BIN 3", "Nominal.BIN 4", "Nominal.BIN 5", "Nominal.BIN 6", "Nominal.BIN 7", "Nominal.BIN 8", "Nominal.BIN 9", "Nominal.BIN 10": Value Change {
        n435 = event-data() -> ("CtlRef"=→"Nominal REF":refnum<vi>, "NewVal"=→"Nom New Val":dbl)  [unwired: 1 in, 4 out]
        n436 = call-poly "Enqueue Message.vi"("Message"="LowNominal", "Message Queue"=w1179) -> ("dup Message Queue"=w1178:refnum<queue>)  [unwired: 8 in, 1 out]
      }
      event "% Tolerance.BIN 1", "% Tolerance.BIN 2", "% Tolerance.BIN 3", "% Tolerance.BIN 4", "% Tolerance.BIN 5", "% Tolerance.BIN 6", "% Tolerance.BIN 7", "% Tolerance.BIN 8", "% Tolerance.BIN 9", "% Tolerance.BIN 10": Value Change {
        n437 = event-data() -> ("CtlRef"=→"% Tolerance Ref":refnum<vi>, "NewVal"=→"Tolerance New Val":dbl)  [unwired: 1 in, 4 out]
        n438 = call-poly "Enqueue Message.vi"("Message"="UpperTol", "Message Queue"=w1184) -> ("dup Message Queue"=w1183:refnum<queue>)  [unwired: 8 in, 1 out]
      }
      event "COMP State", "Comparator Beeper", "Comparator Mode", "Comparator Clear", "Comparator Upper", "Comparator Lower": Value Change {
        n439 = event-data() -> ("CtlRef"=→"COMP Ref":refnum<vi>)  [unwired: 1 in, 5 out]
        n440 = call-poly "Enqueue Message.vi"("Message"="Configure Comparator", "Message Queue"=w1189) -> ("dup Message Queue"=w1188:refnum<queue>)  [unwired: 8 in, 1 out]
      }
      event "BIN No..BIN 1", "BIN No..BIN 2", "BIN No..BIN 3", "BIN No..BIN 4", "BIN No..BIN 5", "BIN No..BIN 6", "BIN No..BIN 7", "BIN No..BIN 8", "BIN No..BIN 9", "BIN No..BIN 10": Value Change {
        n441 = event-data() -> ("CtlRef"=→"BIN NO. Ref":refnum<vi>, "NewVal"=→"BIN No.State":bool)  [unwired: 1 in, 4 out]
        n442 = call-poly "Enqueue Message.vi"("Message"="BIN State", "Message Queue"=w1193) -> ("dup Message Queue"=w1192:refnum<queue>)  [unwired: 8 in, 1 out]
      }
      event "Settings": Value Change {
        n443 = event-data() -> ()  [unwired: 1 in, 1 out]
        n444 = call-poly "Enqueue Message.vi"("Message"="Launch Settings Dialog", "Message Queue"=w1197) -> ("dup Message Queue"=w1196:refnum<queue>)  [unwired: 8 in, 1 out]
      }
      event "Stop": Value Change {
        n445 = event-data() -> ()  [unwired: 1 in, 1 out]
        n446 = call-poly "Enqueue Message.vi"("Message"="Stop", "Message Queue"=w1201) -> ("error out"=w1200:errorcluster, "dup Message Queue"=w1199:refnum<queue>)  [unwired: 8 in]
      }
      event "Disconnect": Value Change {
        n447 = event-data() -> ()  [unwired: 1 in, 1 out]
        n448 = call-poly "Enqueue Message.vi"("Message"="Disconnect", "Message Queue"=w1205) -> ("dup Message Queue"=w1204:refnum<queue>)  [unwired: 8 in, 1 out]
      }
      event Panel Close? {
        # "Send the 'Confirm Quit' message if the user closes the panel of the VI. Discard the event so the 'Confirm Quit' message has a chance to run."
        n449 = event-data() -> ()  [unwired: 1 in, 1 out]
        n450 = call-poly "Enqueue Message.vi"("Priority Message? (F)"=TRUE, "Message"="Confirm Quit", "Message Queue"=w1209) -> ("error out"=w1207:errorcluster, "dup Message Queue"=w1208:refnum<queue>)  [unwired: 7 in]
        n451 = event-data("Discard?"=TRUE) -> ()  [unwired: 1 in, 1 out]
      }
      event Application Instance Close {
        n452 = event-data() -> ()  [unwired: 1 in, 1 out]
      }
      event "Exit": Value Change {
        w1215 = TRUE  # Priority Message
        # "The UI Message Loop handles sending the Exit message to other loops."
        n453 = event-data() -> ()  [unwired: 1 in, 1 out]
        n454 = call-poly "Enqueue Message.vi"("Priority Message? (F)"=w1215, "Message"="Exit", "Message Queue"=w1214) -> ("error out"=w1217:errorcluster, "dup Message Queue"=w1213:refnum<queue>)  [unwired: 7 in]
      }
      event User Event {
        # "The Message Handling Loop processed an \"Exit\" message, which fired this event to stop the Event Handling Loop."
        n455 = event-data() -> ()  [unwired: 1 in, 1 out]
        n456 = local write "Status"("Exit" ("Exit String")) -> ()
      }
    }
    n457 = call "Error Handler - Event Handling Loop.vi"("error in (no error)"=w1143, "Message Queue"=w1142) -> ("dup error in"=w1144:errorcluster)  [unwired: 8 in, 1 out]
  }
  n458 = while "Data Display Loop" {
    tunnel: w13 -> [w1225]
    stop <- w1226 stop-if-true
    # "Data Display Loop"
    n459 = Wait on Notification(notifier=w1225) -> (notification=w1224:T4, error out=w1226:errorcluster)  [unwired: 3 in, 2 out]
    n460 = Unbundle By Name(w1224) -> ("Function"=→"Function":string, "Resistance"=→"Res":dbl, "Temp"=→"Temp":dbl)
  }
  n461 = Obtain Notifier(notification data type="Stat In") -> (notifier out=w3:refnum<notifier>)  [unwired: 3 in, 2 out]
  n462 = while "Data Display Loop" {
    tunnel: w3 -> [w1244]
    stop <- w1243 stop-if-true
    # "Stat Display Loop"
    n463 = Wait on Notification(notifier=w1244) -> (notification=w1242:T1, error out=w1243:errorcluster)  [unwired: 3 in, 2 out]
    n464 = Unbundle By Name(w1242) -> ("Sample Count"=→"Sample Count":i32, "IN Sample Count"=→"In Samlpe Count":i32, "Mean"=→"Mean":dbl, "MAX"=→"MAX":dbl, "MAX Index"=→"MAX Index":i32, "MIN"=→"MIN":dbl, "MIN Index"=→"MIN Index":i32, "HIGH"=→"HIGH":i32, "IN"=→"IN":i32, "LOW"=→"LOW":i32, "MEAS Error"=→"MEAS Error":i32, "Deviation"=→"Deviation":dbl, "Variance"=→"Variance":dbl, "Cp"=→"Cp":dbl, "CpK"=→"Cpk":i32)
  }
  n465 = Obtain Notifier(notification data type=w10) -> (notifier out=w5:refnum<notifier>)  [unwired: 3 in, 2 out]
  n466 = while "Data Display Loop" {
    tunnel: w5 -> [w1252]
    stop <- w1251 stop-if-true
    # "COMP Data Display Loop"
    n467 = Wait on Notification(notifier=w1252) -> (notification=w1250:T5, error out=w1251:errorcluster)  [unwired: 3 in, 2 out]
    n468 = Unbundle By Name(w1250) -> ("Result"=→"Comp":string, "Total"=→"TOT :":i32, "IN"=→"IN :":i32, "High"=→"HI :":i32, "Low"=→"LO :":i32)
  }
  n469 = Unregister For Events(event registration refnum=w28, error in=w35) -> (error out=w29:errorcluster)
  n470 = Release Queue(queue=w17, error in (no error)=w36) -> (error out=w24:errorcluster)  [unwired: 1 in, 2 out]
  n471 = Obtain Notifier(notification data type=0 ("BIN Result")) -> (notifier out=w4:refnum<notifier>)  [unwired: 3 in, 2 out]
  n472 = call "Acquisition Message Loop.vi"("Comp Notifier"=w5, "BIN Notifier"=w4, "Stat Notifier"=w3, "error in (no error)"=w30, "Meas Queue"=w12, "Meas Notifier"=w13, "Message Queues"=w32) -> ("error out"=w34:errorcluster)  [unwired: 4 in]
  n473 = Release Queue(queue=w12, error in (no error)=w24) -> (error out=w23:errorcluster)  [unwired: 1 in, 2 out]
  n474 = Release Notifier(notifier=w13, error in (no error)=w23) -> (error out=w9:errorcluster)  [unwired: 1 in, 2 out]
  n475 = while "Data Display Loop" {
    tunnel: w4 -> [w1260]
    stop <- w1261 stop-if-true
    # "BIN Data Display Loop"
    n476 = Wait on Notification(notifier=w1260) -> (notification=w1259:i32, error out=w1261:errorcluster)  [unwired: 3 in, 2 out]
    n477 = property on="BIN Display" class="Clust (strict)"() -> ("Controls[]"=w1253:refnum<vi>[])  [unwired: 2 in, 2 out]
    n478 = Logarithm Base 2(1:w1259) -> (0:w1256:dbl)
    n479 = Index Array(array=w1253, index=w1256) -> (element=w1258:refnum<vi>)
    n480 = Delete From Array(array=w1253, length=1, index=w1256) -> (array with subset deleted=w1254:refnum<vi>[])  [unwired: 1 out]
    n481 = property class="Ctl"(reference=w1258, "Value"=TRUE) -> ()  [unwired: 1 in, 2 out]
    n482 = for {
      tunnel: w1254 -> [w1262] mode=indexing
      n483 = property class="Ctl"(reference=w1262, "Value"=FALSE) -> ()  [unwired: 1 in, 2 out]
    }
  }
  n484 = Release Notifier(notifier=w3, error in (no error)=w9) -> (error out=w8:errorcluster)  [unwired: 1 in, 2 out]
  n485 = Release Notifier(notifier=w5, error in (no error)=w8) -> (error out=w7:errorcluster)  [unwired: 1 in, 2 out]
  n486 = Release Notifier(notifier=w4, error in (no error)=w7) -> (error out=w6:errorcluster)  [unwired: 1 in, 2 out]
  n487 = Merge Errors(w29, w6, w34, w31) -> (w26:errorcluster)
  n488 = call "Destroy User Event - Stop.vi"("error in (no error)"=w26, "User Event - Stop"=w21) -> ("error out"=w25:errorcluster)  [unwired: 9 in]
  n489 = disable-structure shown="RUN_TIME_ENGINE==True" {
    disable-tunnel: w25 -> [_ _]
    frame condition #0 (active) {
    }
    frame condition #1 {
      # "Call Quit LabVIEW if running as a built application."
      n490 = Quit LabVIEW() -> ()  [unwired: 1 in]
    }
  }
